vi "MTS_Main.vi"() -> ()   [LabVIEW 2010]
panel:
  out "Counts":u32[](array[numeric])
  in  "Autopoint-Auto Z":bool=TRUE
  in  "psf width [um]":dbl=0.7
  out "Last Image File No":i32
  out "NxtAutMesPoint":i32
  out "Auto Measure Points":i32
  out "Pattern":dbl[][](array[numeric])
  out "Active pt3":path
  in  "Axis":enum32{"x-y", "x-z", "y-z"}(ring)
  in  "Save Files":bool=TRUE
  out "Intensity (a.u.)":dbl=1.0 format="%.02f"
  out "Detector2":bool
  out "Detector1":bool
  out "Excitation":bool
  in  "Measurement Time (ms)":i32=60000 min=10
  in  "Open MSW":bool
  in  "New MSW":bool
  out "Workspace":path
  in  "WS File Tree":string(tree)
  out "Stop Measurement":bool
  in  "Learning loop":bool=TRUE
  in  "ShowTab":T1(tab)=enum."TCSPC Histogram"
  out "Video":u8[][](graph)
  in  "Find Mols":bool
  out "Image":i32[][](graph)
  in  "Save Color Image":bool
  out "Auto Meas Progress":i32(slide) caption="Point 1 / 1" scale=0.0..1.0
  out "AM image":T2(plugin-control)
  in  "Auto Meas":bool
  in  "Auto Measurement Time (ms)":i32=10000 caption="Measurement Time (ms)" min=10
  out "Histogram":i32[][](graph)
  out "Trace":i32[][](graph)
  out "FiFo Overrun":bool
  in  "SCANNER EMERGENCY":bool
  out "Measure. time [s]":i32
  in  "Scanner Divider":i32=2 min=1 max=10
  out "y":dbl format="%.1f nm"
  out "x":dbl format="%.1f nm"
  in  "x-Pixel":u16=100
  in  "y-Pixel":u16=100
  in  "Picture size":dbl=50.0 min=0.1 max=200.0 format="%1.1f um"
  in  "Picture size 2":dbl=50.0 min=0.1 max=200.0 format="%1.1f um"
  in  "Z-Position":dbl=50.0 caption="Z" min=0.0 max=200.0 format="%1.3f um"
  in  "Y-Position":dbl=50.0 caption="Y" min=0.0 max=200.0 format="%1.3f um"
  in  "X-Position":dbl=50.0 caption="X" min=0.0 max=200.0 format="%1.3f um"
  out "Do Measurement":T3(ring)
  in  "Point Measurement":bool
  in  "Aquire Image":bool
  in  "Settings":bool
  in  "PI E710 Port":u16(ring) items=["COM1", "COM2", "COM3", "COM4", "COM5", "COM6", "COM7", "COM8", "COM9"]
  in  "Move Stage":bool
  out "MeasRunig":bool
  in  "Stop Program":bool
  out "Global Stop":bool
  # "Workspace"
  # "Shutter:"
  # "Image Scan Settings"
  # "Point Measurement Settings"
  # "upper left corner/ Point Position"
  # "Auto Measurement Settings"
  # "Pixelsize"
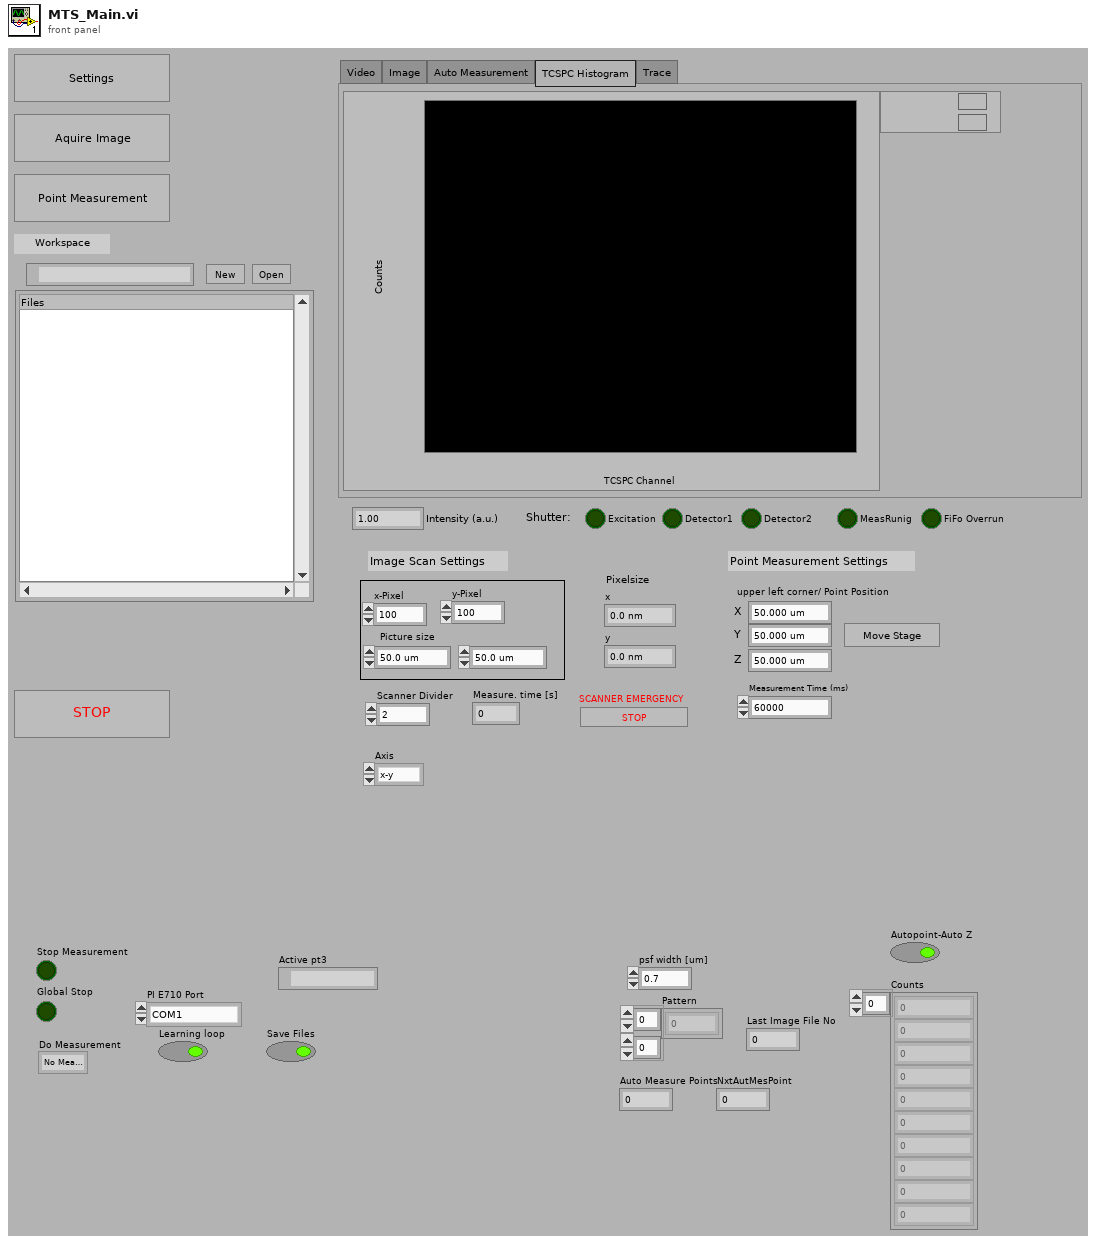
[diagram p1: front panel]
types:
  T1 = enum32{"Video", "Image", "Auto Measurement", "TCSPC Histogram", "Trace"}
  T2 = typedef "IMAQ Image.ctl" = refnum<image>
  T3 = enum16{"No Measurement", "Aquire Image", "Point Measurement", "Multi Measurement", "Save Color Image", "Find Single Mol.", "Auto Measurement Control", "Auto Point"}
  T4 = enum16{"CAN_Baud_1M", "CAN_BAUD_500K", "CAN_BAUD_250K", "CAN_BAUD_125K", "CAN_BAUD_100K", "CAN_BAUD_50K", "CAN_BAUD_20K", "CAN_BAUD_10K", "CAN_BAUD_5K", "User"}
  T5 = enum16{"No Measurement", "Aquire Image", "Point Measurement", "Multi Measurement"}
  T6 = typedef "Image Type" = u32
  T7 = cluster{"Height":u32, "Width":u32, "Pixel Depth":u32}
  T8 = cluster{"Dev":i32, "SerNo":string, "HW_Model":string, "HW_Version":string}[]
  T9 = enum32{"Video", "Image", "TCSPC Histogram", "Trace"}
  T10 = cluster{"ID":u32, "MSG type":enum8{"STD, NO RTR", "STD,RTR", "XTD, NO RTR", "XTD, RTR"}, "LEN":u8, "DATA":u8[]}
  T11 = enum16{"No Measurement", "Aquire Image", "Point Measurement", "Multi Measurement", "Save Color Image"}
  T12 = enum16{"No Measurement", "Aquire Image", "Point Measurement", "Multi Measurement", "Save Color Image", "Find Single Mol."}
  T13 = enum16{"Get (Default)", "Set Workspace", "Append File", "Change Comment"}
  T14 = enum16{"unknown", "pt3 File", "png Image", "bmp Image"}
  T15 = cluster{"File No":i32, "File Path":path, "Parent File":i32, "File Type":enum16{"unknown", "pt3 File", "png Image", "bmp Image"}, "Measurement Type":enum16{"not a pt3 File", "Image File", "Point Measurement", "Auto Point"}, "Upper Left":cluster{"x-Position":dbl, "y-Position":dbl, "z-Position":dbl}, "Pixels":i32[], "Picture Size":dbl[], "Scan Axis":enum32{"x-y", "x-z", "y-z"}}[]
  T16 = typedef "LVPoint32TypeDef.ctl" = cluster{"Horizontal":i32, "Vertical":i32}
  T17 = cluster{"Shift":bool, "Ctrl":bool, "Alt":bool, "Cmd":bool, "Opt":bool}
  T18 = cluster{"File No":i32, "File Path":path, "Parent File":i32, "File Type":enum16{"unknown", "pt3 File", "png Image", "bmp Image"}, "Measurement Type":enum16{"not a pt3 File", "Image File", "Point Measurement", "Auto Point"}, "Upper Left":cluster{"x-Position":dbl, "y-Position":dbl, "z-Position":dbl}, "Pixels":i32[], "Picture Size":dbl[], "Scan Axis":enum32{"x-y", "x-z", "y-z"}}
  T19 = enum16{"not a pt3 File", "Image File", "Point Measurement", "Auto Point"}
  T20 = cluster{"x-Position":dbl, "y-Position":dbl, "z-Position":dbl}
  T21 = cluster{"ID":u32, "MSG type":enum8{"STD, NO RTR", "STD,RTR", "XTD, NO RTR", "XTD, RTR"}, "LEN":u8, "Data":u8[]}
  T22 = cluster{"X-Position":dbl, "Y-Position":dbl, "Z-Position":dbl}
  T23 = cluster{"Dimensions":i32, "Time Per Pixel [ms]":dbl, "Acceleration":i32, "Pattern":i32, "X0":sgl, "Y0":sgl, "PixX":i32, "PixY":i32, "PixResol":sgl, "TStartTo":sgl, "TStoptTo":sgl, "TStartFro":sgl, "TStopFro":sgl}
  T24 = cluster{"Picture Size":dbl[], "Pixels":i32[], "Upper Left":cluster{"x-Position":dbl, "y-Position":dbl, "z-Position":dbl}}
  T25 = cluster{"Dev":i32, "SerNo":string, "HW_Model":string, "HW_Version":string}
  T26 = cluster{"Comment":string, "RangeNo":i32, "Offset":i32, "AcquisitionTime (ms)":i32, "HardwareSerial":i32, "SyncDivider":i32, "Resolution (ns)":sgl, "CFD Settings":cluster{"Ch0 Level":i32, "Ch0 ZeroX":i32, "Ch1 Level":i32, "Ch1 ZeroX":i32}, "InpRate0":i32, "InpRate1":i32}
  T27 = cluster{"Ident":string, "Format Version":string, "Creator Name":string, "Creator Version":string, "File Time":string, "Comment":string, "RangeNo":i32, "Offset":i32, "AcquisitionTime (ms)":i32, "HardwareSerial":i32, "SyncDivider":i32, "Resolution (ns)":sgl, "CFD Settings":cluster{"Ch0 Level":i32, "Ch0 ZeroX":i32, "Ch1 Level":i32, "Ch1 ZeroX":i32}, "InpRate0":i32, "InpRate1":i32}
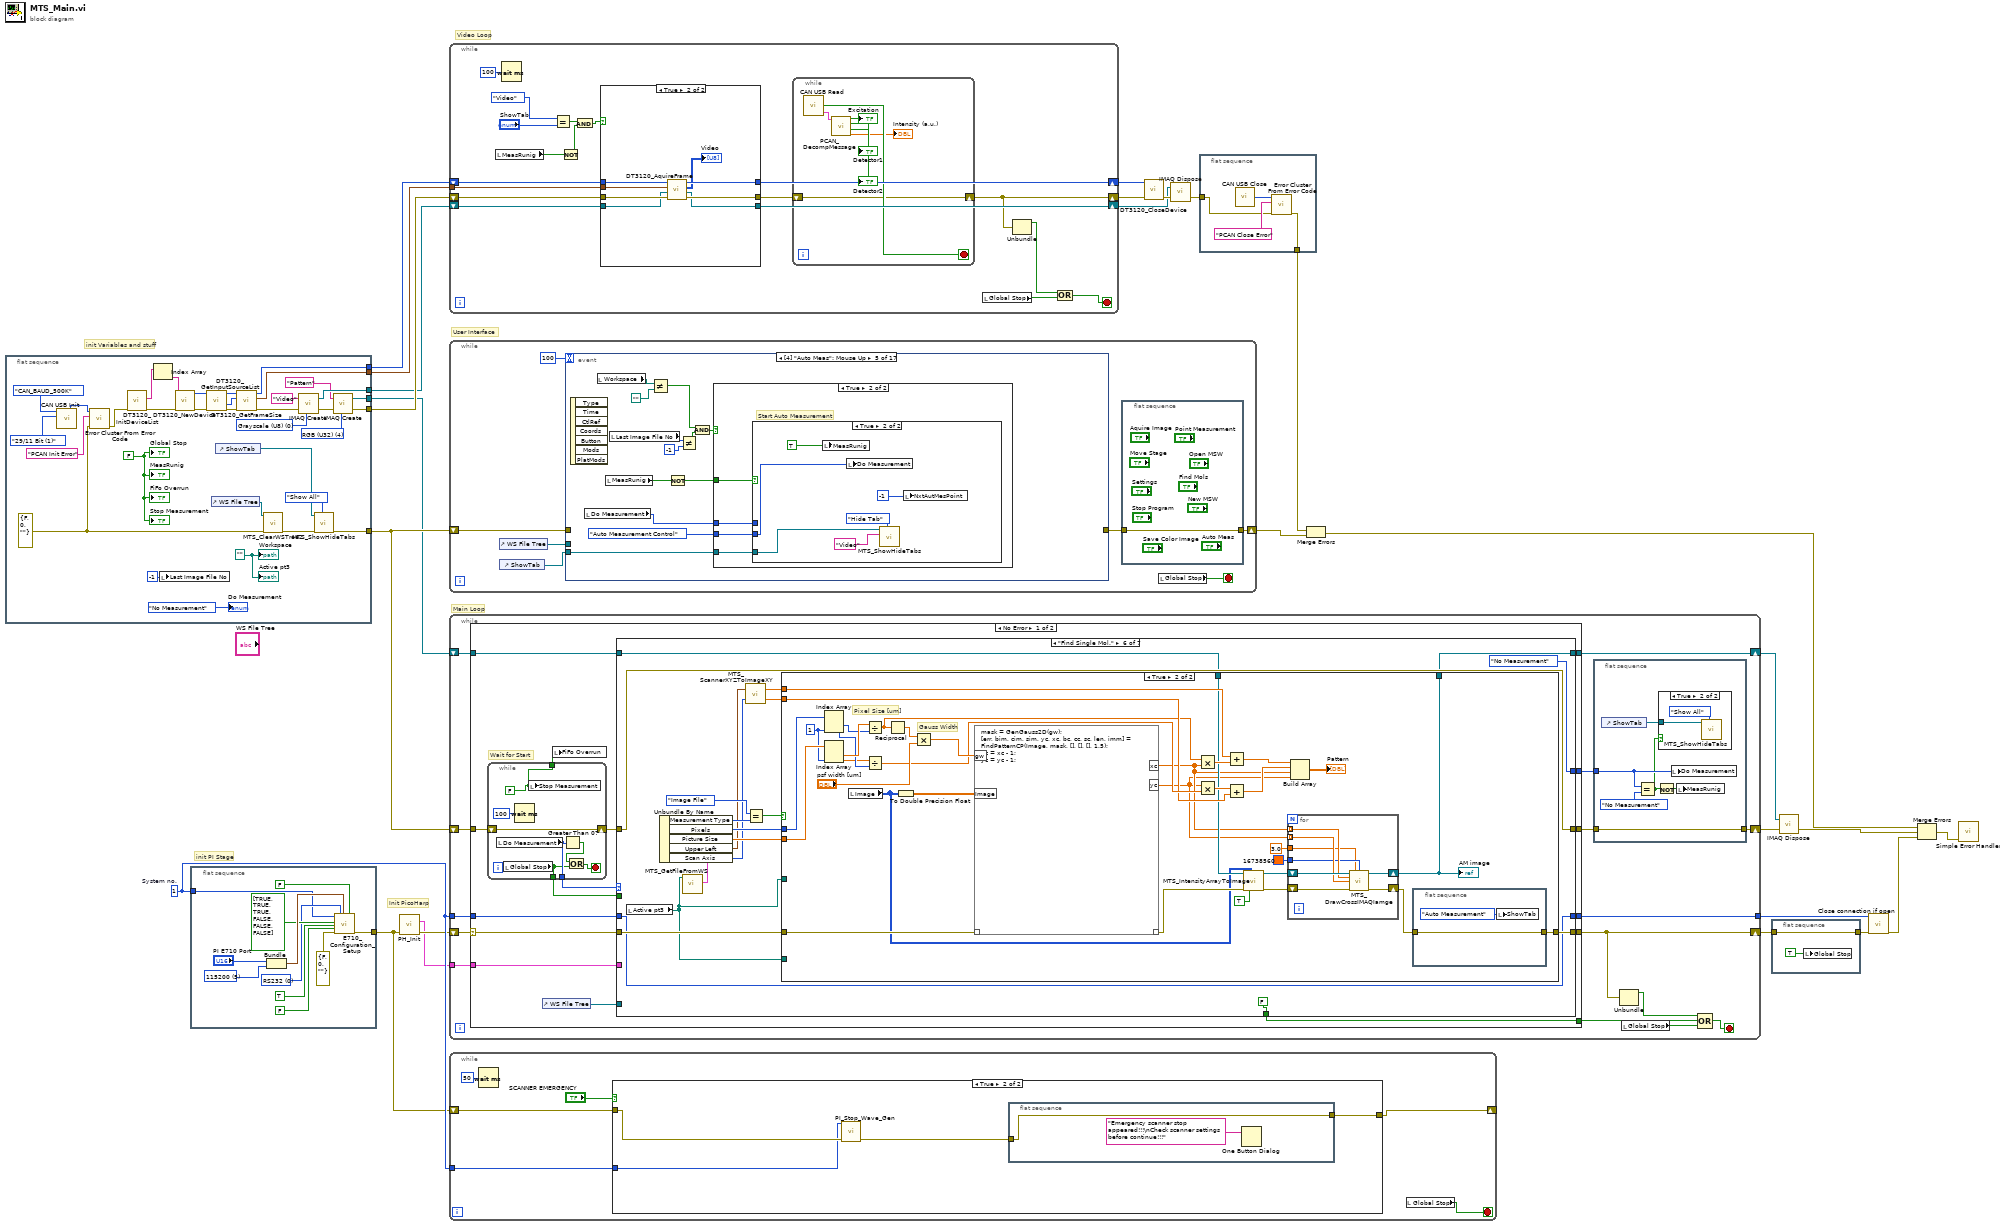
[diagram p0: block diagram]
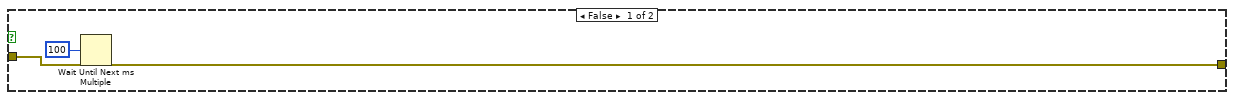
[diagram p3: hidden frame]
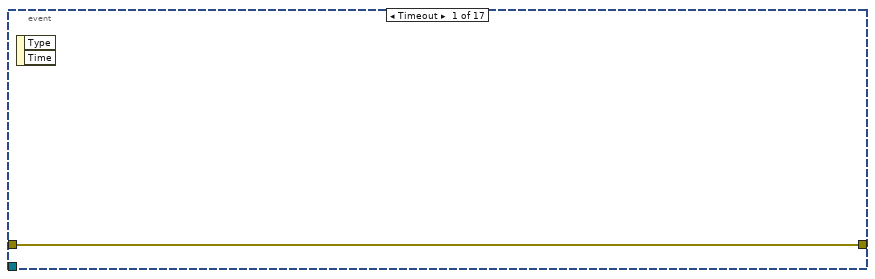
[diagram p4: hidden frame]
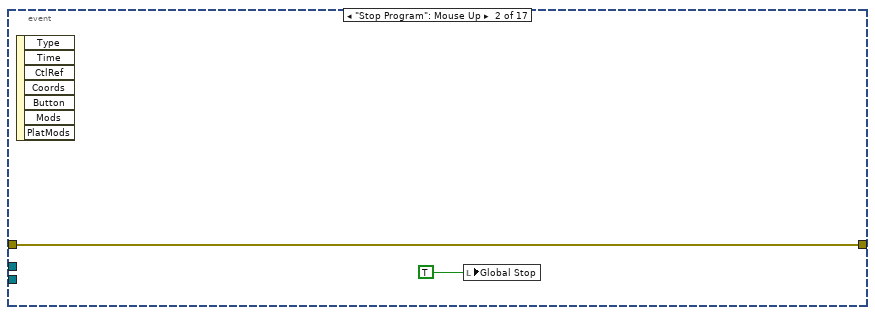
[diagram p5: hidden frame]
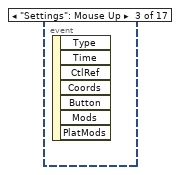
[diagram p6: hidden frame]
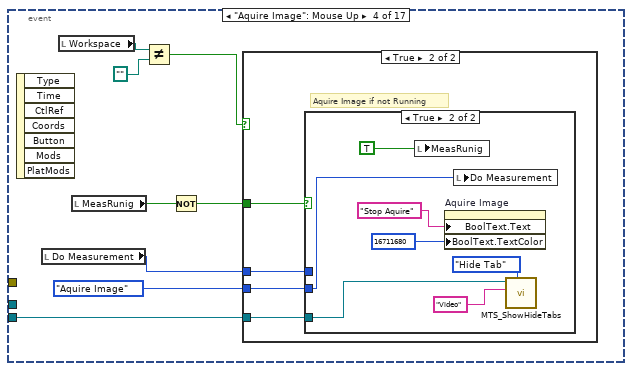
[diagram p7: hidden frame]
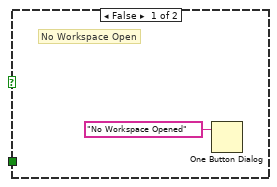
[diagram p8: hidden frame]
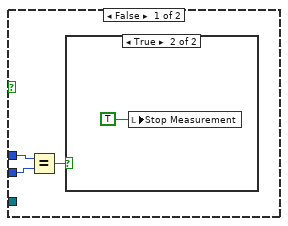
[diagram p9: hidden frame]
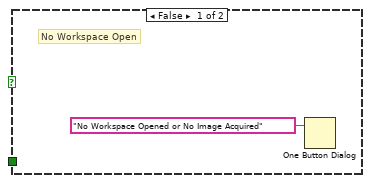
[diagram p11: hidden frame]
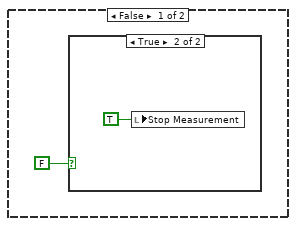
[diagram p12: hidden frame]
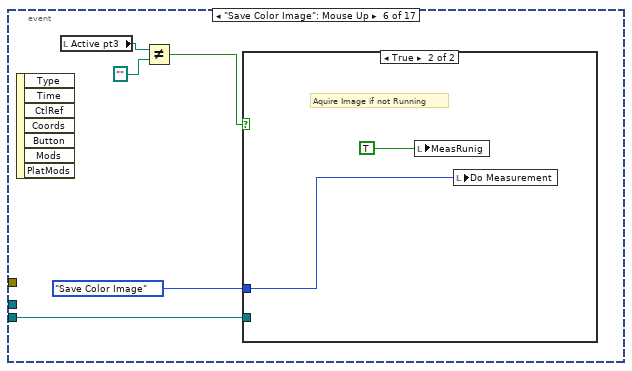
[diagram p14: hidden frame]
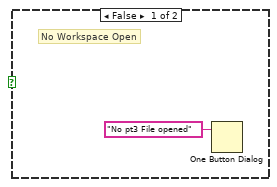
[diagram p15: hidden frame]
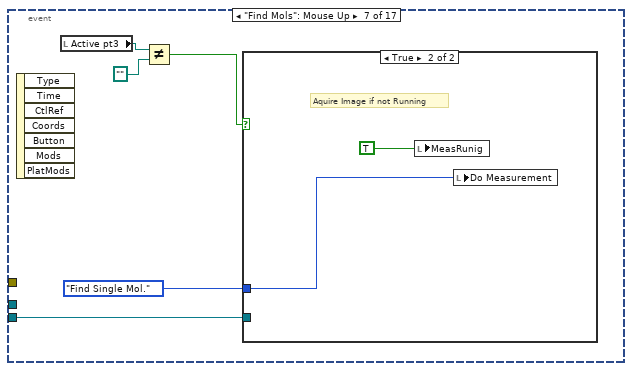
[diagram p16: hidden frame]
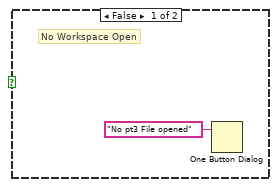
[diagram p17: hidden frame]
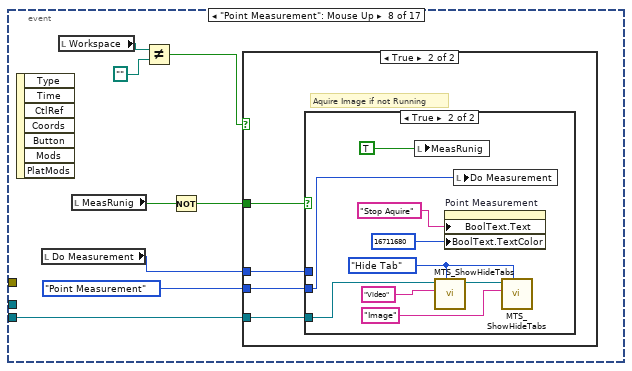
[diagram p18: hidden frame]
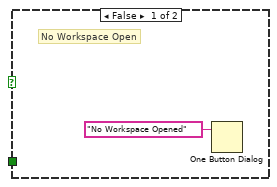
[diagram p19: hidden frame]
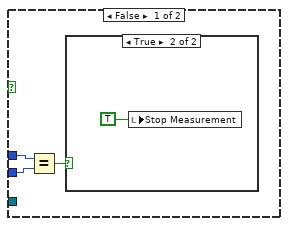
[diagram p20: hidden frame]
diagram:
  w22 = 1  # System no.
  # "Video Loop"
  # "Init PicoHarp"
  # "init Variables and stuff"
  # "User Interface"
  # "init PI Stage"
  # "Main Loop"
  n1 = flat-sequence {
    tunnel: [w43] -> w23
    tunnel: [w32] -> w16
    tunnel: [w50] -> w14
    tunnel: [w47] -> w10
    tunnel: [w31] -> w9
    tunnel: [w28] -> w1
    frame #0 {
      w29 = T6 4 items=["Grayscale (U8)", "Grayscale (I16)", "Grayscale (SGL)", "Complex (CSG)", "RGB (U32)", "HSL (U32)", "RGB (U64)", "Grayscale (U16)"] ("Image Type")
      w48 = T6 0 items=["Grayscale (U8)", "Grayscale (I16)", "Grayscale (SGL)", "Complex (CSG)", "RGB (U32)", "HSL (U32)", "RGB (U64)", "Grayscale (U16)"] ("Image Type")
      w34 = path ""
      w37 = errorcluster {"status"=FALSE, "code"=0, "source"=""} ("error in")
      w59 = FALSE ("Global Stop")
      n2 = call "CAN USB Init.vi"("CAN Msg Type"=enum16{"11 Bit (0)", "29/11 Bit (1)"}."29/11 Bit (1)", "BTR0BTR1"=T4."CAN_BAUD_500K") -> ("Error Number"=w38:u32)  [unwired: 7 in, 2 out]
      n3 = call <vilib>:"Error Cluster From Error Code.vi"("error in (no error)"=w37, "error message (\"\")"="PCAN Init Error" ("error message (\"\")"), "error code (0)"=w38) -> ("error out"=w36:errorcluster)  [unwired: 6 in]
      n4 = call "DT3120_InitDeviceList.vi"("error in (no error)"=w36) -> ("error out"=w57:errorcluster, "Alias List"=w58:string[])  [unwired: 9 out]
      n5 = Index Array(array=w58) -> (element=w56:string)  [unwired: 1 in]
      n6 = local write "Last Image File No"(-1 ("Last Image File No")) -> ()
      n7 = call "DT3120_NewDevice.vi"("error in (no error)"=w57, "Alias"=w56) -> ("error out"=w52:errorcluster, "DevId"=w51:i32)  [unwired: 8 out]
      n8 = call "DT3120_GetInputSourceList.vi"("error in (no error)"=w52, "DevId"=w51) -> ("error out"=w55:errorcluster, "Active Source"=w54:u16, "DevId (dup)"=w53:i32)  [unwired: 7 out]
      n9 = control-ref of="WS File Tree"() -> (w45:refnum<vi>)
      n10 = control-ref of="ShowTab"() -> (w42:refnum<vi>)
      n11 = call "DT3120_GetFrameSize.vi"("error in (no error)"=w55, "Source"=w54, "DevId"=w53) -> ("error out"=w49:errorcluster, "Frame Size"=w47:T7, "DevId (dup)"=w50:i32)  [unwired: 6 in]
      n12 = call "MTS_ClearWSTree2.vi"("error in"=w37, "Tree Refnum"=w45) -> ("error out"=w44:errorcluster)  [unwired: 8 in, 1 out]
      n13 = call "IMAQ Create"("Image Name"="Video", "Image Type"=w48, "error in (no error)"=w49) -> ("New Image"=w31:T2, "error out"=w33:errorcluster)  [unwired: 2 in]
      n14 = call "MTS_ShowHideTabs.vi"("Action"=enum16{"Show All", "Hide Tab", "Show Tab"}."Show All", "error in (no error)"=w44, "ShowTab"=w42) -> ("error out"=w43:errorcluster)  [unwired: 7 in, 1 out]
      n15 = call "IMAQ Create"("Image Name"="Pattern", "Image Type"=w29, "error in (no error)"=w33) -> ("New Image"=w28:T2, "error out"=w32:errorcluster)  [unwired: 2 in]
      "Global Stop" <- w59
      "MeasRunig" <- w59
      "Do Measurement" <- T5."No Measurement" ("Do Measurement")
      "FiFo Overrun" <- w59
      "Stop Measurement" <- w59
      "Workspace" <- w34
      "Active pt3" <- w34
    }
  }
  n16 = flat-sequence {
    tunnel: [w63] -> w21
    tunnel: w22 -> [w62]
    frame #0 {
      w70 = u16 5 items=["9600", "14400", "19200", "38400", "57600", "115200"] ("Baudrate")
      w65 = u16 0 items=["RS232", "GPIB"] ("Interface")
      n17 = Bundle("PI E710 Port"="PI E710 Port", "Baudrate"=w70) -> (w71:cluster{"PI E710 Port":u16, "Baudrate":u16})  [unwired: 1 out]
      n18 = call <userlib>:"E710_Configuration_Setup.vi"("System no."=w62, "Are stages connected?"=bool[] [TRUE, TRUE, TRUE, FALSE, FALSE, FALSE], "Change servo \nstatus to ON?"=TRUE ("Change servo \nstatus to ON?"), "Perform autozero?"=FALSE ("All axes?"), "error in"=errorcluster {"status"=FALSE, "code"=0, "source"=""}, "Interface"=w65, "RS232 settings"=w71, "Move to middle?"=FALSE) -> ("error out"=w63:errorcluster)  [unwired: 4 in, 7 out]
    }
  }
  n19 = call "PH_Init.vi"("error in (no error)"=w21) -> ("Device List"=w19:T8, "error out"=w20:errorcluster)  [unwired: 12 in, 1 out]
  n20 = while {
    shift-right: [w72] -> w15
    shift-left: w16 -> [w86]
    shift-right: [w79] -> w13
    shift-left: w14 -> [w80]
    tunnel: w10 -> [w81]
    shift-right: [w78] -> w7
    shift-left: w9 -> [w82]
    stop <- w85 stop-if-true
    n21 = local read "MeasRunig"() -> (w77:bool)
    n22 = Wait (ms)(milliseconds to wait=u32 100) -> ()  [unwired: 1 out]
    n23 = Equal?(x=T9."Video" ("ShowTab"), y="ShowTab") -> (x = y?=w76:bool)
    n24 = Not(x=w77) -> (.not. x?=w74:bool)
    n25 = And(x=w76, y=w74) -> (x .and. y?=w75:bool)
    n26 = case shown="True" w75 {
      tunnel: w86 -> [w99 w107]
      tunnel: [w99 w106] -> w73
      tunnel: w82 -> [w97 w105]
      tunnel: w81 -> [_ w104]
      tunnel: w80 -> [w98 w103]
      tunnel: [w98 w102] -> w79
      tunnel: [w97 w101] -> w78
      frame False {
      }
      frame True {
        n27 = call "DT3120_AquireFrame.vi"("error in (no error)"=w107, "Image"=w105, "Frame Size"=w104, "DevId"=w103) -> ("error out"=w106:errorcluster, "Image Out"=w101:T2, "Frame"=→"Video":u8[][], "DevId (dup)"=w102:i32)  [unwired: 4 in]
      }
    }
    n28 = while {
      shift-right: [w91] -> w72
      shift-left: w73 -> [w91]
      stop <- w96 stop-if-true
      n29 = call "CAN USB Read.vi"() -> ("RcvQueueEmpty"=w96:bool, "CAN_Message out"=w95:T10)  [unwired: 1 in, 1 out]
      n30 = call "PCAN_DecompMessage.vi"("CAN_Message out"=w95) -> ("Intensity (a.u.)"=→"Intensity (a.u.)":dbl, "Detector2 Shutter Open?"=→"Detector2":bool, "Detector1 Shutter Open?"=→"Detector1":bool, "Excitation Shutter Open?"=→"Excitation":bool)  [unwired: 7 in]
    }
    n31 = local read "Global Stop"() -> (w84:bool)
    n32 = Unbundle(w72) -> ("status"=w83:bool)  [unwired: 2 out]
    n33 = Compound Arithmetic op=OR(w83, w84) -> (w85:bool)
  }
  n34 = while {
    shift-right: [w112] -> w12
    shift-left: w23 -> [w113]
    stop <- w110 stop-if-true
    n35 = control-ref of="WS File Tree"() -> (w109:refnum<vi>)
    n36 = control-ref of="ShowTab"() -> (w108:refnum<vi>)
    n37 = event shown="[4] \"Auto Meas\": Mouse Up" {
      selector: _ -> [_ _ _ _ _ _ _ _ _ _ _ _ _ _ _ _ _]
      dyn-events: _ -> [_ _ _ _ _ _ _ _ _ _ _ _ _ _ _ _ _]
      timeout: 100 -> [_ _ _ _ _ _ _ _ _ _ _ _ _ _ _ _ _]
      tunnel: w113 -> [w116 w118 _ _ _ _ _ _ _ w227 w263 _ w315 _ _ _ _]
      tunnel: [w116 w118 _ _ _ _ _ _ _ w225 w260 _ w314 _ _ _ _] -> w111
      tunnel: w109 -> [_ _ _ _ _ _ _ _ _ w229 w264 _ _ _ _ _ _]
      tunnel: w108 -> [_ _ _ w119 w149 w168 w176 w184 w210 _ _ _ _ _ _ _ _]
      event Timeout {
        n38 = event-data() -> ()  [unwired: 1 in, 2 out]
      }
      event "Stop Program": Mouse Up {
        n39 = event-data() -> ()  [unwired: 1 in, 7 out]
        n40 = local write "Global Stop"(TRUE ("Global Stop")) -> ()
      }
      event "Settings": Mouse Up {
        n41 = event-data() -> ()  [unwired: 1 in, 7 out]
      }
      event "Aquire Image": Mouse Up {
        n42 = event-data() -> ()  [unwired: 1 in, 7 out]
        n43 = local read "Do Measurement"() -> (w123:T3)
        n44 = local read "Workspace"() -> (w122:path)
        n45 = local read "MeasRunig"() -> (w126:bool)
        n46 = Not Equal?(x=w122, y=path "") -> (x != y?=w120:bool)
        n47 = Not(x=w126) -> (.not. x?=w125:bool)
        n48 = case shown="True" w120 {
          tunnel: w125 -> [_ w131]
          tunnel: T11."Aquire Image" ("Do Measurement") -> [_ w130]
          tunnel: w123 -> [_ w129]
          tunnel: w119 -> [_ w128]
          frame False {
            # "No Workspace Open"
            n49 = One Button Dialog(message="No Workspace Opened") -> ()  [unwired: 1 in, 1 out]
          }
          frame True {
            # "Aquire Image if not Running"
            n50 = case shown="True" w131 {
              tunnel: w130 -> [w133 w140]
              tunnel: w129 -> [w134 _]
              tunnel: w128 -> [_ w136]
              frame False {
                n51 = Equal?(x=w134, y=w133) -> (x = y?=w132:bool)
                n52 = case shown="True" w132 {
                  frame False {
                  }
                  frame True {
                    n53 = local write "Stop Measurement"(TRUE ("Stop Measurement")) -> ()
                  }
                }
              }
              frame True {
                n54 = local write "MeasRunig"(TRUE ("Measurement Running")) -> ()
                n55 = property on="Aquire Image" class="Bool"("BoolText.Text"="Stop Aquire" ("Caption.Text"), "BoolText.TextColor"=u32 16711680 ("Boolean Text.Colors:FG Color")) -> ()  [unwired: 2 in, 2 out]
                n56 = local write "Do Measurement"(w140) -> ()
                n57 = call "MTS_ShowHideTabs.vi"("Action"=enum16{"Show All", "Hide Tab", "Show Tab"}."Hide Tab", "Tab Caption"="Video", "ShowTab"=w136) -> ()  [unwired: 7 in, 2 out]
              }
            }
          }
        }
      }
      event "Auto Meas": Mouse Up {
        n58 = event-data() -> ()  [unwired: 1 in, 7 out]
        n59 = local read "Do Measurement"() -> (w152:T3)
        n60 = local read "Workspace"() -> (w151:path)
        n61 = local read "MeasRunig"() -> (w154:bool)
        n62 = local read "Last Image File No"() -> (w147:i32)
        n63 = Not Equal?(x=w151, y=path "") -> (x != y?=w145:bool)
        n64 = Not(x=w154) -> (.not. x?=w153:bool)
        n65 = Not Equal?(x=w147, y=-1) -> (x != y?=w144:bool)
        n66 = And(x=w145, y=w144) -> (x .and. y?=w143:bool)
        n67 = case shown="True" w143 {
          tunnel: w153 -> [_ w159]
          tunnel: T3."Auto Measurement Control" ("Do Measurement") -> [_ w158]
          tunnel: w152 -> [_ w157]
          tunnel: w149 -> [_ w156]
          frame False {
            # "No Workspace Open"
            n68 = One Button Dialog(message="No Workspace Opened or No Image Acquired") -> ()  [unwired: 1 in, 1 out]
          }
          frame True {
            # "Start Auto Measurement"
            n69 = case shown="True" w159 {
              tunnel: w158 -> [_ w166]
              tunnel: w157 -> [_ _]
              tunnel: w156 -> [_ w163]
              frame False {
                n70 = case shown="True" FALSE {
                  frame False {
                  }
                  frame True {
                    n71 = local write "Stop Measurement"(TRUE ("Stop Measurement")) -> ()
                  }
                }
              }
              frame True {
                n72 = local write "MeasRunig"(TRUE ("Measurement Running")) -> ()
                n73 = local write "Do Measurement"(w166) -> ()
                n74 = call "MTS_ShowHideTabs.vi"("Action"=enum16{"Show All", "Hide Tab", "Show Tab"}."Hide Tab", "Tab Caption"="Video", "ShowTab"=w163) -> ()  [unwired: 7 in, 2 out]
                n75 = local write "NxtAutMesPoint"(-1 ("Next Auto Measure Point")) -> ()
              }
            }
          }
        }
      }
      event "Save Color Image": Mouse Up {
        n76 = event-data() -> ()  [unwired: 1 in, 7 out]
        n77 = local read "Active pt3"() -> (w171:path)
        n78 = Not Equal?(x=w171, y=path "") -> (x != y?=w169:bool)
        n79 = case shown="True" w169 {
          tunnel: T12."Save Color Image" ("Do Measurement") -> [_ w175]
          tunnel: w168 -> [_ _]
          frame False {
            # "No Workspace Open"
            n80 = One Button Dialog(message="No pt3 File opened") -> ()  [unwired: 1 in, 1 out]
          }
          frame True {
            # "Aquire Image if not Running"
            n81 = local write "MeasRunig"(TRUE ("Measurement Running")) -> ()
            n82 = local write "Do Measurement"(w175) -> ()
          }
        }
      }
      event "Find Mols": Mouse Up {
        n83 = event-data() -> ()  [unwired: 1 in, 7 out]
        n84 = local read "Active pt3"() -> (w179:path)
        n85 = Not Equal?(x=w179, y=path "") -> (x != y?=w177:bool)
        n86 = case shown="True" w177 {
          tunnel: T12."Find Single Mol." ("Do Measurement") -> [_ w183]
          tunnel: w176 -> [_ _]
          frame False {
            # "No Workspace Open"
            n87 = One Button Dialog(message="No pt3 File opened") -> ()  [unwired: 1 in, 1 out]
          }
          frame True {
            # "Aquire Image if not Running"
            n88 = local write "MeasRunig"(TRUE ("Measurement Running")) -> ()
            n89 = local write "Do Measurement"(w183) -> ()
          }
        }
      }
      event "Point Measurement": Mouse Up {
        n90 = event-data() -> ()  [unwired: 1 in, 7 out]
        n91 = local read "Do Measurement"() -> (w188:T3)
        n92 = local read "Workspace"() -> (w187:path)
        n93 = local read "MeasRunig"() -> (w191:bool)
        n94 = Not Equal?(x=w187, y=path "") -> (x != y?=w185:bool)
        n95 = Not(x=w191) -> (.not. x?=w190:bool)
        n96 = case shown="True" w185 {
          tunnel: w190 -> [_ w196]
          tunnel: T11."Point Measurement" ("Do Measurement") -> [_ w195]
          tunnel: w188 -> [_ w194]
          tunnel: w184 -> [_ w193]
          frame False {
            # "No Workspace Open"
            n97 = One Button Dialog(message="No Workspace Opened") -> ()  [unwired: 1 in, 1 out]
          }
          frame True {
            # "Aquire Image if not Running"
            n98 = case shown="True" w196 {
              tunnel: w195 -> [w198 w207]
              tunnel: w194 -> [w199 _]
              tunnel: w193 -> [_ w204]
              frame False {
                n99 = Equal?(x=w199, y=w198) -> (x = y?=w197:bool)
                n100 = case shown="True" w197 {
                  frame False {
                  }
                  frame True {
                    n101 = local write "Stop Measurement"(TRUE ("Stop Measurement")) -> ()
                  }
                }
              }
              frame True {
                w201 = enum16{"Show All", "Hide Tab", "Show Tab"}."Hide Tab" ("Action")
                n102 = local write "MeasRunig"(TRUE ("Measurement Running")) -> ()
                n103 = call "MTS_ShowHideTabs.vi"("Action"=w201, "Tab Caption"="Video", "ShowTab"=w204) -> ("ShowTab (dup)"=w203:refnum<vi>)  [unwired: 7 in, 1 out]
                n104 = property on="Point Measurement" class="Bool"("BoolText.Text"="Stop Aquire" ("Caption.Text"), "BoolText.TextColor"=u32 16711680 ("Boolean Text.Colors:FG Color")) -> ()  [unwired: 2 in, 2 out]
                n105 = local write "Do Measurement"(w207) -> ()
                n106 = call "MTS_ShowHideTabs.vi"("Action"=w201, "Tab Caption"="Image", "ShowTab"=w203) -> ()  [unwired: 7 in, 2 out]
              }
            }
          }
        }
      }
      event "Move Stage": Mouse Up {
        n107 = event-data() -> ()  [unwired: 1 in, 7 out]
        n108 = local read "Do Measurement"() -> (w214:T3)
        n109 = local read "Workspace"() -> (w213:path)
        n110 = local read "MeasRunig"() -> (w217:bool)
        n111 = Not Equal?(x=w213, y=path "") -> (x != y?=w211:bool)
        n112 = Not(x=w217) -> (.not. x?=w216:bool)
        n113 = case shown="True" w211 {
          tunnel: w216 -> [_ w222]
          tunnel: T11."Multi Measurement" ("Do Measurement") -> [_ w221]
          tunnel: w214 -> [_ w220]
          tunnel: w210 -> [_ w219]
          frame False {
            # "No Workspace Open"
            n114 = One Button Dialog(message="No Workspace Opened") -> ()  [unwired: 1 in, 1 out]
          }
          frame True {
            # "Aquire Image if not Running"
            n115 = case shown="True" w222 {
              tunnel: w221 -> [_ w223]
              tunnel: w220 -> [_ _]
              tunnel: w219 -> [_ _]
              frame False {
              }
              frame True {
                n116 = local write "MeasRunig"(TRUE ("Measurement Running")) -> ()
                n117 = local write "Do Measurement"(w223) -> ()
              }
            }
          }
        }
      }
      event "New MSW": Mouse Up {
        # "Default Name"
        n118 = event-data() -> ()  [unwired: 1 in, 7 out]
        n119 = flat-sequence {
          tunnel: [w245] -> w228
          tunnel: w227 -> [w245]
          frame #0 {
            n120 = local write "MeasRunig"(TRUE ("MeasRunig")) -> ()
          }
        }
        n121 = Get Date/Time In Seconds() -> (seconds since 1Jan1904=w242:timestamp)
        n122 = Format Date/Time String(time format string (%c)="%Y-%m-%d", seconds (now)=w242) -> (date/time string=w240:string)  [unwired: 1 out]
        n123 = Concatenate Strings(w240, ".msw" ("string")) -> (w238:string)
        n124 = call "File Dialog"("start path"=path "E:/", "prompt"="Create New Workspace", "button label"="Create", "default name"=w238, "error in"=w228, "pattern (all files)"="*.msw", "pattern label"="MT Scan Workspace") -> ("selected path"=w232:path, "cancelled"=w233:bool, "error out"=w231:errorcluster)  [unwired: 5 in, 1 out]
        n125 = case shown="False" w233 {
          tunnel: w232 -> [w251 _]
          tunnel: w231 -> [w257 w259]
          tunnel: [w249 w258] -> w226
          tunnel: w229 -> [w247 _]
          frame False {
            # "Create Empty Workspace"
            n126 = local write "Workspace"(w251) -> ()
            n127 = call "MTS_CreateWriteMSW.vi"("Rewrite"=TRUE, "error in (no error)"=w257, "Workspace Path"=w251) -> ("error out"=w250:errorcluster, "Created"=w254:string, "Comment (dup)"=w253:string, "Files in Workspace (dup)"=w252:T15)  [unwired: 5 in]
            n128 = call "MTS_Workspace.vi"("Workspace"=w251, "Operation"=T13."Set Workspace", "Created in"=w254, "New Comment"=w253, "Files in Workspace in"=w252) -> ("Files in Workspace"=w248:T15)  [unwired: 3 in, 3 out]
            n129 = call "MTS_BuildWSTree.vi"("error in"=w250, "Files in Workspace"=w248, "Tree Refnum"=w247) -> ("error out"=w249:errorcluster)  [unwired: 7 in, 1 out]
          }
          frame True {
            n130 = call <vilib>:"Clear Errors.vi"("error in (no error)"=w259) -> ("error out"=w258:errorcluster)  [unwired: 6 in]
          }
        }
        n131 = flat-sequence {
          tunnel: w226 -> [w243]
          tunnel: [w243] -> w225
          frame #0 {
            n132 = local write "MeasRunig"(FALSE ("MeasRunig")) -> ()
          }
        }
      }
      event "Open MSW": Mouse Up {
        n133 = event-data() -> ()  [unwired: 1 in, 7 out]
        n134 = flat-sequence {
          tunnel: w263 -> [w275]
          tunnel: [w275] -> w262
          frame #0 {
            n135 = local write "MeasRunig"(TRUE ("MeasRunig")) -> ()
          }
        }
        n136 = call "File Dialog2"("start path"=path "E:/", "prompt"="Create New Workspace", "button label"="Open", "error in"=w262, "pattern (all files)"="*.msw", "pattern label"="MT Scan Workspace") -> ("selected path"=w267:path, "cancelled"=w268:bool, "error out"=w266:errorcluster)  [unwired: 6 in, 1 out]
        n137 = case shown="False" w268 {
          tunnel: w267 -> [w281 _]
          tunnel: w266 -> [w286 w288]
          tunnel: [w279 w287] -> w261
          tunnel: w264 -> [w277 _]
          frame False {
            # "Open Workspace"
            n138 = local write "Workspace"(w281) -> ()
            n139 = call "MTS_ReadMSW.vi"("error in (no error)"=w286, "Workspace Path"=w281) -> ("error out"=w280:errorcluster, "Created"=w284:string, "Comment"=w283:string, "Files in Workspace"=w282:T15)  [unwired: 6 in]
            n140 = call "MTS_Workspace.vi"("Workspace"=w281, "Operation"=T13."Set Workspace", "Created in"=w284, "New Comment"=w283, "Files in Workspace in"=w282) -> ("Files in Workspace"=w278:T15)  [unwired: 3 in, 3 out]
            n141 = call "MTS_BuildWSTree.vi"("error in"=w280, "Files in Workspace"=w278, "Tree Refnum"=w277) -> ("error out"=w279:errorcluster)  [unwired: 7 in, 1 out]
          }
          frame True {
            n142 = call <vilib>:"Clear Errors.vi"("error in (no error)"=w288) -> ("error out"=w287:errorcluster)  [unwired: 6 in]
          }
        }
        n143 = flat-sequence {
          tunnel: w261 -> [w273]
          tunnel: [w273] -> w260
          frame #0 {
            n144 = local write "MeasRunig"(FALSE ("MeasRunig")) -> ()
          }
        }
      }
      event "Image": Mouse Up {
        w291 = 100.0 ("y")
        n145 = event-data() -> ("Coords"=w303:T16, "PlatMods"=w304:T17)  [unwired: 1 in, 5 out]
        n146 = local read "Axis"() -> (w299:enum32{"x-y", "x-z", "y-z"})
        n147 = invoke on="Image" class="IntGraph (strict)" method="Map Coords To XY"("Coords"=w303) -> ("Map Coords To XY"=w300:bool, "XY"=w298:cluster{"X":dbl, "Y":dbl})  [unwired: 6 in, 5 out]
        n148 = Unbundle By Name(w304) -> ("Ctrl"=w301:bool)
        n149 = And(x=w300, y=w301) -> (x .and. y?=w302:bool)
        n150 = Unbundle(w298) -> ("X"=w297:dbl, "Y"=w294:dbl)
        n151 = Multiply(x=w297, y=w291) -> (x*y=w296:dbl)
        n152 = Multiply(x=w294, y=w291) -> (x*y=w293:dbl)
        n153 = Round To Nearest(number=w296) -> (nearest integer value=w295:dbl)
        n154 = Round To Nearest(number=w293) -> (nearest integer value=w292:dbl)
        n155 = Divide(x=w295, y=w291) -> (x/y=w290:dbl)
        n156 = Divide(x=w292, y=w291) -> (x/y=w289:dbl)
        n157 = case shown="True" w302 {
          tunnel: w299 -> [_ w307]
          tunnel: w290 -> [_ w306]
          tunnel: w289 -> [_ w305]
          frame False {
          }
          frame True {
            n158 = case shown="\"x-y\", Default" w307 {
              tunnel: w306 -> [w309 w311 w313]
              tunnel: w305 -> [w308 w310 w312]
              frame "x-y", Default {
                n159 = local write "X-Position"(w309) -> ()
                n160 = local write "Y-Position"(w308) -> ()
              }
              frame "x-z" {
                n161 = local write "X-Position"(w311) -> ()
                n162 = local write "Z-Position"(w310) -> ()
              }
              frame "y-z" {
                n163 = local write "Y-Position"(w313) -> ()
                n164 = local write "Z-Position"(w312) -> ()
              }
            }
          }
        }
      }
      event "WS File Tree": Value Change {
        n165 = event-data() -> ("NewVal"=w319:string)  [unwired: 1 in, 4 out]
        n166 = local read "Workspace"() -> (w316:path)
        n167 = Not Equal?(x=w316, y=path "") -> (x != y?=w317:bool)
        n168 = case shown="True" w317 {
          tunnel: w319 -> [_ w330]
          tunnel: w316 -> [_ w329]
          tunnel: w315 -> [w320 w328]
          tunnel: [w320 w327] -> w314
          frame False {
          }
          frame True {
            n169 = call "MTS_GetFileFromWS.vi"("Tree Label"=w330) -> ("File Header"=w326:T18, "File Found"=w325:bool)  [unwired: 9 in]
            n170 = Unbundle By Name(w326) -> ("File Type"=w324:T14)
            n171 = Equal?(x=w324, y=T14."pt3 File" ("File Type")) -> (x = y?=w322:bool)
            n172 = And(x=w325, y=w322) -> (x .and. y?=w321:bool)
            n173 = case shown="True" w321 {
              tunnel: w326 -> [_ w350]
              tunnel: w329 -> [_ w356]
              tunnel: w328 -> [w331 w351]
              tunnel: [w331 w338] -> w327
              frame False {
              }
              frame True {
                # "Image Intensity Array"
                n174 = Unbundle By Name(w350) -> ("Measurement Type"=w337:T19, "Pixels"=w335:i32[], "Picture Size"=w334:dbl[], "Upper Left"=w333:T20, "Scan Axis"=w332:enum32{"x-y", "x-z", "y-z"})
                n175 = Unbundle By Name(w350) -> ("File Path"=w355:path)
                n176 = Strip Path(path=w356) -> (stripped path=w354:path)  [unwired: 1 out]
                n177 = Strip Path(path=w355) -> (name=w353:string)  [unwired: 1 out]
                n178 = control-ref of="Image"() -> (w336:refnum<vi>)
                n179 = Build Path(base path=w354, name or relative path=w353) -> (appended path=w352:path)
                n180 = Index Array(array=w335, index #2=1 ("index")) -> (element #1=w347:i32, element #2=w346:i32)  [unwired: 1 in]
                n181 = local write "Active pt3"(w352) -> ()
                n182 = call "PT3_Open.vi"("error in"=w351, "File Path"=w352) -> ("error out"=w345:errorcluster, "refnum out"=w344:refnum<file>)  [unwired: 3 in, 5 out]
                n183 = Initialize Array(0 ("element"), w347, w346) -> (w343:i32[][])
                n184 = case shown="\"Image File\"" w337 {
                  tunnel: w345 -> [w363 w395]
                  tunnel: w344 -> [w370 w394]
                  tunnel: w343 -> [w369 w393]
                  tunnel: [w367 w392] -> w342
                  tunnel: [w366 w391] -> w341
                  tunnel: [w365 w390] -> w340
                  tunnel: [w364 w389] -> w339
                  tunnel: w336 -> [w361 _]
                  tunnel: w335 -> [w360 _]
                  tunnel: w334 -> [w359 _]
                  tunnel: w333 -> [w358 _]
                  tunnel: w332 -> [w357 _]
                  frame "Image File" {
                    n185 = call "MTS_SetGraphScales.vi"("Pixels"=w360, "Axis"=w357, "Picture Size"=w359, "error in (no error)"=w363, "Upper Left"=w358, "Image"=w361) -> ("error out"=w362:errorcluster)  [unwired: 5 in]
                    n186 = while {
                      tunnel: w370 -> [w385]
                      shift-right: [FALSE ("Start From Top")] -> _
                      shift-left: TRUE ("Start From Top") -> [w379]
                      shift-right: [w378] -> w364
                      shift-left: w362 -> [w374]
                      tunnel: [w377] -> w365
                      tunnel: [w376] -> w367
                      tunnel: [w375] -> w368
                      tunnel: w369 -> [w373]
                      tunnel: [w372] -> w366
                      stop <- w382 stop-if-true
                      n187 = call "PT3_Read.vi"("Start From Top"=w379, "error in"=w374, "Data count"=10000, "refnum in"=w385) -> ("error out"=w378:errorcluster, "Data out"=w381:u32[], "refnum out"=w377:refnum<file>, "EOF?"=w382:bool)  [unwired: 4 in]
                      n188 = Array Size(array=w381) -> (size(s)=w380:i32)
                      n189 = call "MTS_ToImageOffline.vi"("Data In"=w381, "Reset"=w379, "Image Array In"=w373, "Data Count"=w380) -> ("Image Array Out"=w375:i32[][], "Histograms"=w376:i32[][], "Traces"=w372:i32[][])  [unwired: 2 in, 7 out]
                    }
                    n190 = local write "Image"(w368) -> ()
                  }
                  frame "Point Measurement", Default {
                    w396 = TRUE ("Start From Top")
                    n191 = call "PT3_Read.vi"("Start From Top"=w396, "error in"=w395, "Data count"=10000, "refnum in"=w394) -> ("error out"=w389:errorcluster, "Data out"=w387:u32[], "refnum out"=w390:refnum<file>)  [unwired: 4 in, 1 out]
                    n192 = Array Size(array=w387) -> (size(s)=w386:i32)
                    n193 = call "MTS_ToImageOffline.vi"("Data In"=w387, "Reset"=w396, "Image Array In"=w393, "Data Count"=w386) -> ("Histograms"=w392:i32[][], "Traces"=w391:i32[][])  [unwired: 2 in, 8 out]
                  }
                }
                n194 = local write "Histogram"(w342) -> ()
                n195 = local write "Trace"(w341) -> ()
                n196 = Close File(refnum=w340, error in=w339) -> (error out=w338:errorcluster)  [unwired: 1 out]
              }
            }
          }
        }
      }
      event "x-Pixel", "Picture size", "y-Pixel", "Picture size 2": Value Change {
        w399 = 1000.0 ("y")
        n197 = event-data() -> ()  [unwired: 1 in, 5 out]
        n198 = local read "Picture size 2"() -> (w401:dbl)
        n199 = local read "Picture size"() -> (w405:dbl)
        n200 = local read "x-Pixel"() -> (w404:u16)
        n201 = local read "y-Pixel"() -> (w400:u16)
        n202 = Divide(x=w405, y=w404) -> (x/y=w403:dbl)
        n203 = Divide(x=w401, y=w400) -> (x/y=w402:dbl)
        n204 = Multiply(x=w403, y=w399) -> (x*y=→"x":dbl)
        n205 = Multiply(x=w402, y=w399) -> (x*y=→"y":dbl)
      }
      event "Excitation": Mouse Up {
        n206 = event-data() -> ()  [unwired: 1 in, 7 out]
        n207 = local read "MeasRunig"() -> (w407:bool)
        n208 = Not(x=w407) -> (.not. x?=w406:bool)
        n209 = case shown="True" w406 {
          frame False {
          }
          frame True {
            n210 = local read "Excitation"() -> (w411:bool)
            n211 = local read "Detector1"() -> (w409:bool)
            n212 = local read "Detector2"() -> (w408:bool)
            n213 = Not(x=w411) -> (.not. x?=w410:bool)
            n214 = call "PCAN_CompMessage.vi"("Detector2"=w408, "Detector1"=w409, "Excitation"=w410) -> ("CAN_Message"=w412:T21)
            n215 = call "CAN USB Write.vi"("CAN_Message"=w412) -> ()  [unwired: 2 in, 1 out]
          }
        }
      }
      event "Detector1": Mouse Up {
        n216 = event-data() -> ()  [unwired: 1 in, 7 out]
        n217 = local read "MeasRunig"() -> (w414:bool)
        n218 = Not(x=w414) -> (.not. x?=w413:bool)
        n219 = case shown="True" w413 {
          frame False {
          }
          frame True {
            n220 = local read "Excitation"() -> (w415:bool)
            n221 = local read "Detector1"() -> (w417:bool)
            n222 = local read "Detector2"() -> (w418:bool)
            n223 = Not(x=w417) -> (.not. x?=w416:bool)
            n224 = call "PCAN_CompMessage.vi"("Detector2"=w418, "Detector1"=w416, "Excitation"=w415) -> ("CAN_Message"=w419:T21)
            n225 = call "CAN USB Write.vi"("CAN_Message"=w419) -> ()  [unwired: 2 in, 1 out]
          }
        }
      }
      event "Detector2": Mouse Up {
        n226 = event-data() -> ()  [unwired: 1 in, 7 out]
        n227 = local read "MeasRunig"() -> (w421:bool)
        n228 = Not(x=w421) -> (.not. x?=w420:bool)
        n229 = case shown="True" w420 {
          frame False {
          }
          frame True {
            n230 = local read "Excitation"() -> (w425:bool)
            n231 = local read "Detector1"() -> (w424:bool)
            n232 = local read "Detector2"() -> (w422:bool)
            n233 = Not(x=w422) -> (.not. x?=w423:bool)
            n234 = call "PCAN_CompMessage.vi"("Detector2"=w423, "Detector1"=w424, "Excitation"=w425) -> ("CAN_Message"=w426:T21)
            n235 = call "CAN USB Write.vi"("CAN_Message"=w426) -> ()  [unwired: 2 in, 1 out]
          }
        }
      }
    }
    n236 = flat-sequence {
      tunnel: [w115] -> w112
      tunnel: w111 -> [w115]
      frame #0 {
      }
    }
    n237 = local read "Global Stop"() -> (w110:bool)
  }
  n238 = while {
    shift-right: [w432] -> w18
    shift-left: w20 -> [w427]
    tunnel: w22 -> [w440]
    tunnel: [w439] -> w26
    shift-right: [w434] -> w4
    shift-left: w23 -> [w441]
    tunnel: w19 -> [w433]
    shift-right: [w430] -> w2
    shift-left: w1 -> [w429]
    stop <- w437 stop-if-true
    n239 = case shown="No Error" w427 {
      selector: w427 -> [w443 w1032]
      tunnel: w441 -> [w457 w1030]
      tunnel: w440 -> [w456 w1031]
      tunnel: [w455 w1031] -> w439
      tunnel: [w454 TRUE ("Global Stop")] -> w436
      tunnel: [w450 w1030] -> w435
      tunnel: w433 -> [w449 _]
      tunnel: [w448 w1032] -> w432
      tunnel: [w446 w1029] -> w430
      tunnel: w429 -> [w445 w1029]
      tunnel: [w444 T3."No Measurement" ("Do Measurement")] -> w428
      frame No Error {
        # "Wait for Start"
        n240 = while {
          shift-right: [w1026] -> w451
          shift-left: w457 -> [w1026]
          tunnel: [w1023] -> w453
          tunnel: [w1022] -> w452
          tunnel: [w1021] -> w447
          stop <- w1027 stop-if-true
          w1021 = FALSE ("FiFo Overrun")
          n241 = local read "Do Measurement"() -> (w1023:T3)
          n242 = local read "Global Stop"() -> (w1022:bool)
          n243 = Wait (ms)(milliseconds to wait=u32 100) -> ()  [unwired: 1 out]
          n244 = local write "Stop Measurement"(w1021) -> ()
          n245 = Greater Than 0?(x=w1023) -> (x > 0?=w1025:bool)
          n246 = Or(x=w1025, y=w1022) -> (x .or. y?=w1027:bool)
        }
        n247 = control-ref of="WS File Tree"() -> (w442:refnum<vi>)
        n248 = local write "FiFo Overrun"(w447) -> ()
        n249 = case shown="\"Find Single Mol.\"" w453 {
          selector: w453 -> [_ _ w675 _ _ _ _]
          tunnel: w443 -> [w462 w540 w726 w831 w846 w921 w989]
          tunnel: w456 -> [w463 w539 w689 w832 w842 w917 w988]
          tunnel: [w463 w506 w678 w824 w842 w917 w988] -> w455
          tunnel: [w462 w514 w715 w825 w845 w920 w989] -> w448
          tunnel: [w461 FALSE ("Global Stop") FALSE ("Global Stop") FALSE ("Global Stop") FALSE ("Global Stop") FALSE ("Global Stop") FALSE ("Global Stop")] -> w454
          tunnel: w452 -> [w461 _ _ _ _ _ _]
          tunnel: w451 -> [w460 w501 w707 w823 w844 w919 w984]
          tunnel: [w460 w515 w716 w823 w844 w919 w980] -> w450
          tunnel: w449 -> [_ w536 w723 _ _ _ _]
          tunnel: w445 -> [w459 w466 w676 w821 w834 w905 w973]
          tunnel: [w459 w466 w676 w821 w834 w904 w972] -> w446
          tunnel: [T3."No Measurement" ("Do Measurement") T3."No Measurement" ("Do Measurement") w672 T3."No Measurement" ("Do Measurement") T3."No Measurement" ("Do Measurement") T3."No Measurement" ("Do Measurement") w979] -> w444
          tunnel: w442 -> [_ _ w654 _ _ _ _]
          frame "No Measurement", Default {
          }
          frame "Aquire Image" {
            w467 = T19."Image File" ("Measurement Type")
            w513 = 32768 ("dimension size")
            # "TODO:\n- FIFO Read Flag Buffer Half Full?\n- auto square pixels"
            # "Image Intensity Array"
            n250 = control-ref of="Image"() -> (w480:refnum<vi>)
            n251 = Bundle("X-Position"="X-Position", "Y-Position"="Y-Position", "Z-Position"="Z-Position") -> (w476:T22)  [unwired: 1 in]
            n252 = Build Array("x-Pixel", "y-Pixel") -> (w474:u16[])
            n253 = Cluster To Array(cluster=w476) -> (array=w538:dbl[])
            n254 = call "PI_Scanner_In_Range.vi"("Picture size"="Picture size", "Picture size 2"="Picture size 2", "Upper Left"=w476, "Axis"="Axis") -> ("Picture size out"=w500:dbl, "Picture size out 2"=w499:dbl)  [unwired: 14 in]
            n255 = call "PI_MoveTo.vi"("System no."=w539, "Target position"=w538, "error in"=w540, "Move"=TRUE) -> ("System no. (dup)"=w522:i32, "error out"=w479:errorcluster)  [unwired: 13 in, 1 out]
            n256 = Build Array(w500, w499) -> (w475:dbl[])
            n257 = Multiply(x="Scanner Divider", y=2.0) -> (x*y=w469:dbl)
            n258 = call "MTS_SetGraphScales.vi"("Pixels"=w474, "Axis"="Axis", "Picture Size"=w475, "error in (no error)"=w479, "Upper Left"=w476, "Image"=w480) -> ("error out"=w477:errorcluster)  [unwired: 5 in]
            n259 = call "MTS_GenFileComment.vi"("Time Per Pixel [ms]"=w469, "Measurement Type"=w467, "error in"=w501, "Upper Left"=w476, "Pixels"=w474, "Picture Size"=w475) -> ("error out"=w496:errorcluster, "Image Header"=w468:T23, "Image Info"=w486:T24, "Comment"=w498:string)  [unwired: 2 in]
            n260 = local read "Workspace"() -> (w497:path)
            n261 = control-ref of="WS File Tree"() -> (w485:refnum<vi>)
            n262 = call "PI_Image_Scanner_Prepare_Dlg.vi"("System no."=w522, "Picture Size"=w475, "Pixels"=w474, "Axis"="Axis", "Scanner Divider"="Scanner Divider", "error in"=w477, "Learning loop"="Learning loop") -> ("System no. (dup)"=w521:i32, "Measurement time [s]"=w518:i32, "error out"=w523:errorcluster)  [unwired: 6 in]
            n263 = local write "Picture size"(w500) -> ()
            n264 = local write "Picture size 2"(w499) -> ()
            n265 = Index Array(array=w536) -> (element=w535:T25)  [unwired: 1 in]
            n266 = call "MTS_GetNextFileName.vi"("error in (no error)"=w496, "File Type"="pt3", "Measurement Type"="Image", "Workspace"=w497) -> ("error out"=w489:errorcluster, "Next File Name"=w488:path)  [unwired: 6 in]
            n267 = Unbundle By Name(w535) -> ("Dev"=w532:i32)
            n268 = call "PH_Set.vi"("Device List"=w536, "error in (no error)"=w523) -> ("pt3 header out"=w503:T26, "Count Rate"=w525:i32, "error out"=w505:errorcluster)  [unwired: 8 in, 3 out]
            n269 = Initialize Array(0 ("element"), "x-Pixel", "y-Pixel") -> (w526:i32[][])
            n270 = call "MTS_AddFileToWorkspace.vi"("File Name"=w488, "File Type"=T14."pt3 File", "Scan Axis"="Axis", "Measurement Type"=w467, "File Info"=w486, "error in (no error)"=w489, "Tree Refnum"=w485) -> ("File Name (dup)"=w473:path, "File No"=→"Last Image File No":i32, "error out"=w487:errorcluster)  [unwired: 6 in]
            n271 = call "MTS_CalcMeasTime.vi"("Scanner Divider"="Scanner Divider", "pt3 header in"=w503, "Measurement time [s]"=w518, "Count Rate"=w525) -> ("pt3 header out"=w502:T26, "Corrected Measurement time [s]"=→"Measure. time [s]":i32, "Calc Acq. Time (ms)"=w529:i32, "Overflow Interv. Time (s)"=w528:dbl, "Pixel Time (Laser Pulses)"=w524:i32)  [unwired: 7 in]
            n272 = call "PT3_Create.vi"("Image Header in"=w468, "Save pt3"="Save Files", "Measurement Type"=w467, "error in"=w505, "Comment"=w498, "pt3 Header in"=w502, "File Path"=w473) -> ("error out"=w504:errorcluster, "refnum out"=w493:refnum<file>)  [unwired: 3 in]
            n273 = call "PH_Start.vi"("Device Index"=w532, "Acq. Time"=w529, "error in (no error)"=w504) -> ("error out"=w533:errorcluster)  [unwired: 11 in, 1 out]
            n274 = local write "Active pt3"(w473) -> ()
            n275 = To Unsigned Long Integer(number=w513) -> (unsigned 32bit integer=w510:u32)
            n276 = Initialize Array(u32 0, w513) -> (w511:u32[])
            n277 = Unbundle By Name(w533) -> ("status"=w534:bool)
            n278 = Not(x=w534) -> (.not. x?=w531:bool)
            n279 = case shown="True" w531 {
              tunnel: [w594 w621] -> w516
              tunnel: [w596 w613] -> w507
              tunnel: w521 -> [w596 w610]
              tunnel: w533 -> [w595 w611]
              tunnel: w487 -> [w597 w619]
              tunnel: [w597 w618] -> w517
              tunnel: w532 -> [w593 w620]
              tunnel: w528 -> [_ w600]
              tunnel: w526 -> [_ w615]
              tunnel: w524 -> [_ w614]
              tunnel: "Axis" -> [_ w609]
              tunnel: w511 -> [_ w608]
              tunnel: w510 -> [_ w607]
              tunnel: [w592 w606] -> w509
              tunnel: [w592 w605] -> w508
              tunnel: w493 -> [w591 w604]
              tunnel: [w591 w603] -> w492
              tunnel: [0 ("Num Records Total") w602] -> w491
              tunnel: [0.0 w599] -> w490
              tunnel: [u64[] [] ("Histograms") w598] -> w484
              frame False {
                w592 = FALSE ("Stop Measurement")
                n280 = call "PH_Stop.vi"("Device Index"=w593, "error in (no error)"=w595) -> ("error out"=w594:errorcluster)  [unwired: 12 in, 1 out]
              }
              frame True {
                # "Overflow Interv. Time (s)"
                # "No Error"
                n281 = call "PI_Start_Wave_Gen.vi"("System no."=w610, "error in"=w611, "Axis"=w609) -> ("System no. (dup)"=w613:i32, "error out"=w612:errorcluster)  [unwired: 11 in]
                n282 = while {
                  tunnel: w620 -> [w649]
                  tunnel: w608 -> [w648]
                  tunnel: w607 -> [w647]
                  shift-right: [w633] -> w617
                  shift-left: w612 -> [w650]
                  shift-right: [w646] -> w618
                  shift-left: w619 -> [w646]
                  shift-right: [FALSE ("Reset")] -> _
                  shift-left: TRUE ("Reset") -> [w642]
                  tunnel: w615 -> [w639]
                  tunnel: w614 -> [w635]
                  tunnel: [w636] -> w606
                  tunnel: [w626] -> w605
                  tunnel: w604 -> [w630]
                  tunnel: [w629] -> w603
                  tunnel: [w628] -> w602
                  tunnel: [w627] -> w601
                  tunnel: [w622] -> w598
                  stop <- w645 stop-if-true
                  n283 = call "PH_FIFORead.vi"("Device Index"=w649, "Buffer In"=w648, "Count"=w647, "error in (no error)"=w650) -> ("OK"=w637:bool, "Buffer Out"=w631:u32[], "Data Count"=w632:i32, "FiFo Overrun"=w636:bool, "error out"=w634:errorcluster)  [unwired: 7 in]
                  n284 = local write "FiFo Overrun"(w636) -> ()
                  n285 = local read "Global Stop"() -> (w624:bool)
                  n286 = Wait (ms)(milliseconds to wait=u32 10) -> ()  [unwired: 1 out]
                  n287 = Unbundle(w634) -> ("status"=w644:bool)  [unwired: 2 out]
                  n288 = call "PH_ToImage.vi"("Data In"=w631, "Reset"=w642, "Image Array In"=w639, "Data Count"=w632, "Pixel Time (Laser Pulses)"=w635) -> ("Image Array Out"=→"Image":i32[][], "Histograms"=→"Histogram":i32[][], "Total Photon Count"=w622:u64[], "Total Oveflow Count"=w627:u64, "Num Records Total"=w628:i32, "Traces"=→"Trace":i32[][])  [unwired: 4 in, 1 out]
                  n289 = local read "Stop Measurement"() -> (w625:bool)
                  n290 = call "PT3_Write.vi"("error in"=w634, "Data Count"=w632, "Data in"=w631, "refnum in"=w630) -> ("error out"=w633:errorcluster, "refnum out"=w629:refnum<file>)  [unwired: 6 in]
                  n291 = Compound Arithmetic op=OR(invert w637, w644, w624, w625) -> (w645:bool)
                  n292 = Or(x=w625, y=w624) -> (x .or. y?=w626:bool)
                }
                n293 = Multiply(x=w600, y=w601) -> (x*y=w599:dbl)
                n294 = call "PH_Stop.vi"("Device Index"=w620, "error in (no error)"=w617) -> ("error out"=w621:errorcluster)  [unwired: 12 in, 1 out]
              }
            }
            n295 = control-ref of="WS File Tree"() -> (w482:refnum<vi>)
            n296 = flat-sequence {
              tunnel: w517 -> [w576]
              tunnel: w516 -> [w572]
              tunnel: [w576] -> w515
              tunnel: [w550] -> w514
              tunnel: w509 -> [w574]
              tunnel: w508 -> [w561]
              tunnel: w507 -> [w571]
              tunnel: [w570] -> w506
              tunnel: w492 -> [w567]
              tunnel: w491 -> [w566]
              tunnel: w490 -> [w559]
              tunnel: w484 -> [w560]
              tunnel: "Save Files" -> [w549]
              tunnel: w473 -> [w548]
              tunnel: w482 -> [w547]
              frame #0 {
                # "Count Rate (per s)"
                # "Stop WaveGen\nif Aborted"
                # "Finish after Aquire Image"
                n297 = Or(x=w561, y=w574) -> (x .or. y?=w573:bool)
                n298 = case shown="False" w573 {
                  tunnel: w572 -> [w579 w587]
                  tunnel: w571 -> [w578 w586]
                  tunnel: [w578 w585] -> w570
                  tunnel: [w579 w584] -> w568
                  tunnel: [enum16{"timeover", "manual", "overflow"}."timeover" ("Stop Reason") w582] -> w562
                  tunnel: w561 -> [_ w580]
                  frame False {
                  }
                  frame True {
                    n299 = call "PI_Stop_Wave_Gen.vi"("System no."=w586, "error in"=w587) -> ("System no. (dup)"=w585:i32, "error out"=w584:errorcluster)  [unwired: 12 in]
                    n300 = Select(t=enum16{"timeover", "manual", "overflow"}."manual" ("Stop Reason"), s=w580, f=enum16{"timeover", "manual", "overflow"}."overflow" ("Stop Reason")) -> (s? t:f=w582:enum16{"timeover", "manual", "overflow"})
                  }
                }
                n301 = Multiply(x=w559, y=1000.0) -> (x*y=w564:dbl)
                n302 = Divide(x=w560, y=w559) -> (x/y=w558:dbl[])
                n303 = To Long Integer(number=w564) -> (32bit integer=w563:i32)
                n304 = To Long Integer(number=w558) -> (32bit integer=w557:i32[])
                n305 = property on="Aquire Image" class="Bool"("BoolText.Text"="Aquire Image" ("Caption.Text"), "BoolText.TextColor"=u32 0 ("Boolean Text.Colors:FG Color")) -> ()  [unwired: 2 in, 2 out]
                n306 = Index Array(array=w557, index #1=0 ("index"), index #2=1 ("index")) -> (element #1=w554:i32, element #2=w553:i32)
                n307 = local read "Image"() -> (w552:i32[][])
                n308 = call "PT3_Finish.vi"("Input 1 Rate"=w553, "Input 0 Rate"=w554, "Stop Reason"=w562, "error in"=w568, "Num Records"=w566, "Stop After (ms)"=w563, "refnum in"=w567) -> ("error out"=w551:errorcluster)  [unwired: 4 in]
                n309 = call "MTS_SaveImagePng.vi"("Save .png"=w549, "Tree Refnum"=w547, ".pt3 File Name"=w548, "error in"=w551, "Image"=w552) -> ("error out"=w550:errorcluster)  [unwired: 6 in]
              }
            }
          }
          frame "Point Measurement", "Auto Point" {
            w714 = 32768 ("dimension size")
            n310 = local read "Workspace"() -> (w705:path)
            n311 = local read "X-Position"() -> (w692:dbl)
            n312 = local read "Y-Position"() -> (w691:dbl)
            n313 = local read "Z-Position"() -> (w690:dbl)
            n314 = local read "Pattern"() -> (w656:dbl[][])
            n315 = local read "NxtAutMesPoint"() -> (w655:i32)
            n316 = local read "Last Image File No"() -> (w661:i32)
            n317 = Index Array(array=w723) -> (element=w722:T25)  [unwired: 1 in]
            n318 = Bundle("X-Position"=w692, "Y-Position"=w691, "Z-Position"=w690) -> (w658:T22)  [unwired: 1 in]
            n319 = Equal?(x=w675, y=T3."Auto Point" ("Do Measurement")) -> (x = y?=w652:bool)
            n320 = Unbundle By Name(w722) -> ("Dev"=w679:i32)
            n321 = call "MTS_AutoPointCords.vi"("Is Auto Point"=w652, "Cords In"=w658, "Next Auto Measure Point"=w655, "Pattern"=w656) -> ("Cords"=w657:T22)  [unwired: 7 in]
            n322 = Cluster To Array(cluster=w657) -> (array=w725:dbl[])
            n323 = Select(t="Auto Measurement Time (ms)", s=w652, f="Measurement Time (ms)") -> (s? t:f=w662:i32)
            n324 = call "PI_MoveTo.vi"("System no."=w689, "Target position"=w725, "error in"=w726, "Move"=TRUE) -> ("System no. (dup)"=w678:i32, "error out"=w693:errorcluster)  [unwired: 13 in, 1 out]
            n325 = Select(t="AutoPoint" ("Measurement Type"), s=w652, f="Point" ("Measurement Type")) -> (s? t:f=w665:string)
            n326 = Select(t=T19."Auto Point" ("Measurement Type"), s=w652, f=T19."Point Measurement" ("Measurement Type")) -> (s? t:f=w666:T19)
            n327 = Select(t=w661, s=w652, f=-1) -> (s? t:f=w659:i32)
            n328 = call "MTS_GenFileComment.vi"("Parent File No"=w659, "Measurement Type"=w666, "error in"=w707, "Upper Left"=w657) -> ("error out"=w704:errorcluster, "Image Info"=w694:T24, "Comment"=w706:string)  [unwired: 4 in, 1 out]
            n329 = call "PH_Set.vi"("Device List"=w723, "error in (no error)"=w693) -> ("pt3 header out"=w685:T26, "Count Rate"=w686:i32, "error out"=w681:errorcluster)  [unwired: 8 in, 3 out]
            n330 = Bundle By Name(cluster=w685, "AcquisitionTime (ms)"=w662) -> (w684:T26)
            n331 = And(x=w652, y="Autopoint-Auto Z") -> (x .and. y?=w651:bool)
            n332 = Reciprocal(x=w686) -> (1/x=w688:dbl)
            n333 = call "MTS_GetNextFileName.vi"("error in (no error)"=w704, "File Type"="pt3", "Measurement Type"=w665, "Workspace"=w705) -> ("error out"=w698:errorcluster, "Next File Name"=w697:path)  [unwired: 6 in]
            n334 = Scale By Power Of 2(n=16, x=w688) -> (x*2^n=w677:dbl)
            n335 = case shown="True" w651 {
              tunnel: w681 -> [w728 w736]
              tunnel: [w728 w735] -> w680
              tunnel: w679 -> [_ w734]
              tunnel: w678 -> [_ w733]
              tunnel: w677 -> [_ w732]
              tunnel: w657 -> [_ w731]
              frame False {
              }
              frame True {
                # "Auto Z"
                n336 = call "MTS_AutoZPos.vi"("PH Dev"=w734, "OFlow Interv [s]"=w732, "PI System no."=w733, "error in"=w736, "Start Point"=w731) -> ("New Z"=w730:dbl, "Counts"=→"Counts":u32[], "error out"=w735:errorcluster)  [unwired: 8 in]
                n337 = local write "Z-Position"(w730) -> ()
              }
            }
            n338 = call "MTS_AddFileToWorkspace.vi"("File Name"=w697, "File Type"=T14."pt3 File", "Measurement Type"=w666, "File Info"=w694, "error in (no error)"=w698, "Parent"=w659, "Tree Refnum"=w654) -> ("File Name (dup)"=w695:path, "error out"=w696:errorcluster)  [unwired: 6 in, 1 out]
            n339 = call "PT3_Create.vi"("error in"=w680, "Comment"=w706, "pt3 Header in"=w684, "File Path"=w695) -> ("error out"=w708:errorcluster, "refnum out"=w702:refnum<file>)  [unwired: 6 in]
            n340 = call "PH_Start.vi"("Device Index"=w679, "Acq. Time"=w662, "error in (no error)"=w708) -> ("error out"=w720:errorcluster)  [unwired: 11 in, 1 out]
            n341 = To Unsigned Long Integer(number=w714) -> (unsigned 32bit integer=w711:u32)
            n342 = Initialize Array(u32 0, w714) -> (w712:u32[])
            n343 = Unbundle By Name(w720) -> ("status"=w721:bool)
            n344 = Not(x=w721) -> (.not. x?=w719:bool)
            n345 = case shown="True" w719 {
              tunnel: [w773 w793] -> w717
              tunnel: w720 -> [w774 w777]
              tunnel: w696 -> [w775 w791]
              tunnel: [w775 w790] -> w718
              tunnel: w679 -> [w772 w792]
              tunnel: w677 -> [_ w779]
              tunnel: w712 -> [_ w787]
              tunnel: w711 -> [_ w786]
              tunnel: [w771 w785] -> w710
              tunnel: [w771 w784] -> w709
              tunnel: w702 -> [w770 w783]
              tunnel: [w770 w782] -> w701
              tunnel: [0 ("Num Records Total") w781] -> w700
              tunnel: [0.0 w778] -> w699
              tunnel: [u64[] [] ("Total Photon Count") w776] -> w683
              frame False {
                w771 = FALSE ("Stop Measurement")
                n346 = call "PH_Stop.vi"("Device Index"=w772, "error in (no error)"=w774) -> ("error out"=w773:errorcluster)  [unwired: 12 in, 1 out]
              }
              frame True {
                # "Overflow Interv. Time (s)"
                # "No Error"
                n347 = while {
                  tunnel: w792 -> [w818]
                  tunnel: w787 -> [w817]
                  tunnel: w786 -> [w816]
                  shift-right: [w806] -> w789
                  shift-left: w777 -> [w819]
                  shift-right: [w815] -> w790
                  shift-left: w791 -> [w815]
                  shift-right: [FALSE ("Reset")] -> _
                  shift-left: TRUE ("Reset") -> [w811]
                  tunnel: [w808] -> w785
                  tunnel: [w799] -> w784
                  tunnel: w783 -> [w803]
                  tunnel: [w802] -> w782
                  tunnel: [w801] -> w781
                  tunnel: [w800] -> w780
                  tunnel: [w794] -> w776
                  stop <- w814 stop-if-true
                  n348 = call "PH_FIFORead.vi"("Device Index"=w818, "Buffer In"=w817, "Count"=w816, "error in (no error)"=w819) -> ("OK"=w809:bool, "Buffer Out"=w804:u32[], "Data Count"=w805:i32, "FiFo Overrun"=w808:bool, "error out"=w807:errorcluster)  [unwired: 7 in]
                  n349 = local write "FiFo Overrun"(w808) -> ()
                  n350 = local read "Global Stop"() -> (w797:bool)
                  n351 = Wait (ms)(milliseconds to wait=u32 10) -> ()  [unwired: 1 out]
                  n352 = Unbundle(w807) -> ("status"=w813:bool)  [unwired: 2 out]
                  n353 = call "PH_TraceAndHisto.vi"("Data In"=w804, "Reset"=w811, "Data Count"=w805) -> ("Histograms"=w796:i32[][], "Total Photon Count"=w794:u64[], "Total Oveflow Count"=w800:u64, "Num Records Total"=w801:i32, "Traces"=w795:i32[][])  [unwired: 8 in]
                  n354 = local read "Stop Measurement"() -> (w798:bool)
                  n355 = call "PT3_Write.vi"("error in"=w807, "Data Count"=w805, "Data in"=w804, "refnum in"=w803) -> ("error out"=w806:errorcluster, "refnum out"=w802:refnum<file>)  [unwired: 6 in]
                  n356 = local write "Histogram"(w796) -> ()
                  n357 = local write "Trace"(w795) -> ()
                  n358 = Compound Arithmetic op=OR(invert w809, w813, w797, w798) -> (w814:bool)
                  n359 = Or(x=w798, y=w797) -> (x .or. y?=w799:bool)
                }
                n360 = Multiply(x=w779, y=w780) -> (x*y=w778:dbl)
                n361 = call "PH_Stop.vi"("Device Index"=w792, "error in (no error)"=w789) -> ("error out"=w793:errorcluster)  [unwired: 12 in, 1 out]
              }
            }
            n362 = flat-sequence {
              tunnel: w718 -> [w759]
              tunnel: w717 -> [w755]
              tunnel: [w759] -> w716
              tunnel: [w752] -> w715
              tunnel: w710 -> [w757]
              tunnel: w709 -> [w745]
              tunnel: w701 -> [w751]
              tunnel: w700 -> [w750]
              tunnel: w699 -> [w740]
              tunnel: w683 -> [w739]
              frame #0 {
                # "Finish after Measurement"
                n363 = Or(x=w745, y=w757) -> (x .or. y?=w756:bool)
                n364 = case shown="True" w756 {
                  tunnel: w755 -> [w761 w762]
                  tunnel: [w761 w762] -> w753
                  tunnel: [enum16{"timeover", "manual", "overflow"}."timeover" ("Stop Reason") w765] -> w746
                  tunnel: w745 -> [_ w763]
                  frame False {
                  }
                  frame True {
                    n365 = Select(t=enum16{"timeover", "manual", "overflow"}."manual" ("Stop Reason"), s=w763, f=enum16{"timeover", "manual", "overflow"}."overflow" ("Stop Reason")) -> (s? t:f=w765:enum16{"timeover", "manual", "overflow"})
                  }
                }
                n366 = Multiply(x=w740, y=1000.0) -> (x*y=w748:dbl)
                n367 = Divide(x=w739, y=w740) -> (x/y=w741:dbl[])
                n368 = To Long Integer(number=w748) -> (32bit integer=w747:i32)
                n369 = To Long Integer(number=w741) -> (32bit integer=w742:i32[])
                n370 = property on="Point Measurement" class="Bool"("BoolText.Text"="Point Measurement" ("Caption.Text"), "BoolText.TextColor"=u32 0 ("Boolean Text.Colors:FG Color")) -> ()  [unwired: 2 in, 2 out]
                n371 = Index Array(array=w742, index #1=0 ("index"), index #2=1 ("index")) -> (element #1=w738:i32, element #2=w737:i32)
                n372 = call "PT3_Finish.vi"("Input 1 Rate"=w737, "Input 0 Rate"=w738, "Stop Reason"=w746, "error in"=w753, "Num Records"=w750, "Stop After (ms)"=w747, "refnum in"=w751) -> ("error out"=w752:errorcluster)  [unwired: 4 in]
              }
            }
            n373 = Select(t=T3."Auto Measurement Control" ("Do Measurement"), s=w652, f=T3."No Measurement" ("Do Measurement")) -> (s? t:f=w672:T3)
          }
          frame "Multi Measurement" {
            n374 = local read "X-Position"() -> (w830:dbl)
            n375 = local read "Y-Position"() -> (w829:dbl)
            n376 = local read "Z-Position"() -> (w828:dbl)
            n377 = Build Array(w830, w829, w828) -> (w827:dbl[])
            n378 = call "PI_MoveTo.vi"("System no."=w832, "Target position"=w827, "error in"=w831, "Move"=TRUE) -> ("System no. (dup)"=w824:i32, "error out"=w825:errorcluster)  [unwired: 13 in, 1 out]
          }
          frame "Save Color Image" {
            n379 = local read "Active pt3"() -> (w840:path)
            n380 = call "MTS_GetFileFromWS.vi"(".pt3 File Name"=w840) -> ("File Header"=w839:T18)  [unwired: 9 in, 1 out]
            n381 = Unbundle By Name(w839) -> ("Measurement Type"=w838:T19, "Pixels"=w835:i32[])
            n382 = Equal?(x=T19."Image File" ("Measurement Type"), y=w838) -> (x = y?=w836:bool)
            n383 = control-ref of="WS File Tree"() -> (w841:refnum<vi>)
            n384 = case shown="True" w836 {
              tunnel: w846 -> [w847 w876]
              tunnel: w840 -> [_ w875]
              tunnel: w840 -> [_ w858]
              tunnel: [w847 w848] -> w845
              tunnel: w841 -> [_ w855]
              tunnel: w835 -> [_ w854]
              frame False {
              }
              frame True {
                # "Image Intensity Array"
                # "Image Intensity Array"
                n385 = call "PT3_Open.vi"("error in"=w876, "File Path"=w875) -> ("error out"=w868:errorcluster, "Header"=w872:T27, "refnum out"=w874:refnum<file>)  [unwired: 3 in, 4 out]
                n386 = Index Array(array=w854, index #2=1 ("index")) -> (element #1=w851:i32, element #2=w852:i32)  [unwired: 1 in]
                n387 = Unbundle By Name(w872) -> ()  [unwired: 15 out]
                n388 = Initialize Array(0 ("element"), w851, w852) -> (w870:i32[][])
                n389 = while {
                  tunnel: w874 -> [w902]
                  shift-right: [FALSE ("Start From Top")] -> _
                  shift-left: TRUE ("Start From Top") -> [w896]
                  shift-right: [w895] -> w867
                  shift-left: w868 -> [w890]
                  tunnel: [w894] -> w866
                  tunnel: w870 -> [w893]
                  tunnel: [w892] -> w869
                  tunnel: [w891] -> _
                  stop <- w899 stop-if-true
                  n390 = call "PT3_Read.vi"("Start From Top"=w896, "error in"=w890, "Data count"=10000, "refnum in"=w902) -> ("error out"=w895:errorcluster, "Data out"=w898:u32[], "refnum out"=w894:refnum<file>, "EOF?"=w899:bool)  [unwired: 4 in]
                  n391 = Array Size(array=w898) -> (size(s)=w897:i32)
                  n392 = call "MTS_ToImageOffline.vi"("Data In"=w898, "Reset"=w896, "Image Array In"=w893, "Data Count"=w897) -> ("Image Array Out"=w891:i32[][], "Histograms"=w892:i32[][])  [unwired: 2 in, 8 out]
                }
                n393 = call "MTS_SelectTCSPCBinning.vi"("Histograms in"=w869) -> ("TCSPC Binning"=w862:i32[][], "Colors"=w856:u32[], "Active"=w857:bool[])  [unwired: 1 in, 7 out]
                n394 = Initialize Array(0 ("element"), 4 ("dimension size"), w851, w852) -> (w863:i32[][][])
                n395 = while {
                  tunnel: w866 -> [w889]
                  shift-right: [FALSE ("Start From Top")] -> _
                  shift-left: TRUE ("Start From Top") -> [w883]
                  shift-right: [w882] -> w860
                  shift-left: w867 -> [w878]
                  tunnel: [w881] -> w849
                  tunnel: w863 -> [w880]
                  tunnel: [w879] -> w859
                  tunnel: w862 -> [w877]
                  stop <- w886 stop-if-true
                  n396 = call "PT3_Read.vi"("Start From Top"=w883, "error in"=w878, "Data count"=10000, "refnum in"=w889) -> ("error out"=w882:errorcluster, "Data out"=w885:u32[], "refnum out"=w881:refnum<file>, "EOF?"=w886:bool)  [unwired: 4 out]
                  n397 = Array Size(array=w885) -> (size(s)=w884:i32)
                  n398 = call "MTS_ToColorImage.vi"("Data In"=w885, "Reset"=w883, "Image Array In"=w880, "Data Count"=w884, "TCSPC Binning"=w877) -> ("Image Array Out"=w879:i32[][][])  [unwired: 2 in, 8 out]
                }
                n399 = call "MTS_SaveColorImagePng.vi"("Tree Refnum"=w855, ".pt3 File Name"=w858, "error in"=w860, "Colors"=w856, "Active"=w857, "Image"=w859) -> ("error out"=w850:errorcluster)  [unwired: 5 in]
                n400 = Close File(refnum=w849, error in=w850) -> (error out=w848:errorcluster)  [unwired: 1 out]
              }
            }
          }
          frame "Find Single Mol." {
            n401 = local read "Active pt3"() -> (w916:path)
            n402 = call "MTS_GetFileFromWS.vi"(".pt3 File Name"=w916) -> ("File Header"=w915:T18)  [unwired: 9 in, 1 out]
            n403 = Unbundle By Name(w915) -> ("Measurement Type"=w914:T19, "Pixels"=w911:i32[], "Picture Size"=w910:dbl[], "Upper Left"=w909:T20, "Scan Axis"=w908:enum32{"x-y", "x-z", "y-z"})
            n404 = call "MTS_ScannerXYZToImageXY.vi"("Axis"=w908, "Scanner XYZ"=w909) -> ("Image Y"=w906:dbl, "Image X"=w907:dbl)
            n405 = Equal?(x=T19."Image File" ("Measurement Type"), y=w914) -> (x = y?=w912:bool)
            n406 = case shown="True" w912 {
              tunnel: w921 -> [w923 w950]
              tunnel: w916 -> [_ _]
              tunnel: w916 -> [_ _]
              tunnel: [w923 w924] -> w920
              tunnel: w911 -> [_ w957]
              tunnel: w910 -> [_ w956]
              tunnel: w907 -> [_ w944]
              tunnel: w906 -> [_ w945]
              tunnel: w905 -> [w922 w938]
              tunnel: [w922 w933] -> w904
              frame False {
              }
              frame True {
                w955 = 1 ("index")
                # "Gauss Width"
                # "Pixel Size [um]"
                n407 = Index Array(array=w957, index #2=w955) -> (element #1=w953:i32, element #2=w948:i32)  [unwired: 1 in]
                n408 = Index Array(array=w956, index #2=w955) -> (element #1=w954:dbl, element #2=w947:dbl)  [unwired: 1 in]
                n409 = local read "Image"() -> (w937:i32[][])
                n410 = Divide(x=w954, y=w953) -> (x/y=w941:dbl)
                n411 = Divide(x=w947, y=w948) -> (x/y=w946:dbl)
                n412 = Reciprocal(x=w941) -> (1/x=w940:dbl)
                n413 = To Double Precision Float(number=w937) -> (double precision float=w949:dbl[][])
                n414 = Multiply(x=w940, y="psf width [um]") -> (x*y=w951:dbl)
                n415 = script code="mask = GenGauss2D(gw);\n[err, bim, cim, sim, yc, xc, bc, cc, sc, len, imm] = FindPatternCP(Image, mask, [], [], [], 1.5);\nxc = xc - 1;\nyc = yc - 1;"("??"=w950, "gw"=w951, "Image"=w949) -> ("??"=w939:errorcluster, "xc"=w928:dbl[], "yc"=w927:dbl[])
                n416 = Multiply(x=w941, y=w928) -> (x*y=w943:dbl[])
                n417 = Multiply(x=w927, y=w946) -> (x*y=w942:dbl[])
                n418 = Add(x=w944, y=w943) -> (x+y=w930:dbl[])
                n419 = Add(x=w942, y=w945) -> (x+y=w929:dbl[])
                n420 = call "MTS_IntensityArrayToImage.vi"(0:"Image"=w938, 1:"Image"=w937, "error in (no error)"=w939, "Log Scale"=TRUE) -> ("Image Out"=w934:T2, "error out"=w935:errorcluster)  [unwired: 10 in]
                n421 = for {
                  shift-right: [w964] -> w933
                  shift-left: w934 -> [w965]
                  tunnel: w928 -> [w963] mode=indexing
                  tunnel: w927 -> [w962] mode=indexing
                  shift-right: [w966] -> w925
                  shift-left: w935 -> [w967]
                  tunnel: u32 16738560 -> [w961]
                  tunnel: 3.0 ("x") -> [w960]
                  n422 = call "MTS_DrawCrossIMAQIamge.vi"("Image"=w965, "Size"=w960, "Color"=w961, "X"=w963, "Y"=w962, "error in (no error)"=w967) -> ("Image Out"=w964:T2, "error out"=w966:errorcluster)  [unwired: 8 in]
                }
                "AM image" <- w933
                n423 = Build Array(w930, w929, w928, w927) -> (→"Pattern":dbl[][])
                n424 = flat-sequence {
                  tunnel: w925 -> [w958]
                  tunnel: [w958] -> w924
                  frame #0 {
                    n425 = local write "ShowTab"(T1."Auto Measurement" ("ShowTab")) -> ()
                  }
                }
              }
            }
          }
          frame "Auto Measurement Control" {
            # "Init"
            n426 = local read "Pattern"() -> (w978:dbl[][])
            n427 = local read "NxtAutMesPoint"() -> (w971:i32)
            n428 = Index Array(array=w978, index (row)=0) -> (element=w985:dbl[])  [unwired: 1 in]
            n429 = Less Than 0?(x=w971) -> (x < 0?=w983:bool)
            n430 = case shown="True" w983 {
              tunnel: w985 -> [_ w1020]
              tunnel: w984 -> [w1011 w1015]
              tunnel: [w1011 w1014] -> w981
              tunnel: [w1010 w1012] -> w970
              frame False {
                n431 = local read "Auto Measure Points"() -> (w1010:i32)
              }
              frame True {
                n432 = Array Size(array=w1020) -> (size(s)=w1012:i32)
                "Auto Measure Points" <- w1012
                n433 = Number To Decimal String(number=w1012) -> (decimal integer string=w1017:string)  [unwired: 1 in]
                n434 = Concatenate Strings("Point 1 / " ("Caption.Text"), w1017) -> (w1016:string)
                n435 = property on="Auto Meas Progress" class="Slide (strict)"(error in=w1015, "Scale.Minimum"=0.0 ("Scale.Range:Minimum"), "Scale.Maximum"=w1012, "Value"=1 ("Auto Meas Progress"), "Caption.Text"=w1016) -> (error out=w1014:errorcluster)  [unwired: 1 in, 1 out]
              }
            }
            n436 = Increment(x=w971) -> (x+1=w969:i32)
            "NxtAutMesPoint" <- w969
            n437 = Greater Or Equal?(x=w969, y=w970) -> (x >= y?=w982:bool)
            n438 = Increment(x=w969) -> (x+1=w968:i32)
            n439 = Index Array(array=w978, index (row) #1=2 ("index (row)"), index (col) #1=w969, index (row) #2=3 ("index (row)"), index (col) #2=w969) -> (element #1=w975:dbl, element #2=w974:dbl)
            n440 = case shown="True" w982 {
              tunnel: w981 -> [w1000 w1009]
              tunnel: [w1006 w1009] -> w980
              tunnel: [T3."Auto Point" ("Do Measurement") T3."No Measurement" ("Do Measurement")] -> w979
              tunnel: w968 -> [w1001 _]
              tunnel: w975 -> [w998 _]
              tunnel: w974 -> [w997 _]
              tunnel: w973 -> [w994 w1007]
              tunnel: [w993 w1007] -> w972
              tunnel: w970 -> [w990 _]
              frame False {
                # "Prpare For Next Point"
                n441 = call "MTS_DrawCrossIMAQIamge.vi"("Image"=w994, "Size"=3.0 ("x"), "Color"=u32 6618880, "X"=w998, "Y"=w997, "error in (no error)"=w1000) -> ("Image Out"=w993:T2, "error out"=w999:errorcluster)  [unwired: 8 in]
                n442 = Number To Decimal String(number=w990) -> (decimal integer string=w991:string)  [unwired: 1 in]
                n443 = Number To Decimal String(number=w1001) -> (decimal integer string=w1003:string)  [unwired: 1 in]
                n444 = Concatenate Strings("Point " ("Caption.Text"), w1003, " / " ("Caption.Text"), w991) -> (w1002:string)
                n445 = property on="Auto Meas Progress" class="Slide (strict)"(error in=w999, "Value"=w1001, "Caption.Text"=w1002) -> (error out=w1006:errorcluster)  [unwired: 1 in, 1 out]
                n446 = local write "AM image"(w993) -> ()
              }
              frame True {
                # "No More Points"
              }
            }
          }
        }
      }
      frame Error {
      }
    }
    n447 = flat-sequence {
      tunnel: w435 -> [w1039]
      tunnel: [w1039] -> w434
      tunnel: w428 -> [w1035]
      frame #0 {
        n448 = control-ref of="ShowTab"() -> (w1038:refnum<vi>)
        n449 = Equal?(x=w1035, y=T3."No Measurement" ("Do Measurement")) -> (x = y?=w1034:bool)
        n450 = Not(x=w1034) -> (.not. x?=w1037:bool)
        n451 = case shown="True" w1034 {
          tunnel: w1038 -> [_ w1040]
          frame False {
          }
          frame True {
            n452 = call "MTS_ShowHideTabs.vi"("Action"=enum16{"Show All", "Hide Tab", "Show Tab"}."Show All", "ShowTab"=w1040) -> ()  [unwired: 8 in, 2 out]
          }
        }
        n453 = local write "Do Measurement"(w1035) -> ()
        n454 = local write "MeasRunig"(w1037) -> ()
      }
    }
    n455 = Unbundle(w432) -> ("status"=w431:bool)  [unwired: 2 out]
    n456 = local read "Global Stop"() -> (w438:bool)
    n457 = Compound Arithmetic op=OR(w431, w436, w438) -> (w437:bool)
  }
  n458 = while {
    tunnel: w22 -> [w1045]
    shift-right: [w1044] -> _
    shift-left: w21 -> [w1046]
    stop <- w1043 stop-if-true
    n459 = Wait (ms)(milliseconds to wait=u32 50) -> ()  [unwired: 1 out]
    n460 = case shown="True" "SCANNER EMERGENCY" {
      tunnel: w1045 -> [_ w1051]
      tunnel: w1046 -> [w1049 w1052]
      tunnel: [w1049 w1053] -> w1044
      frame False {
        n461 = Wait Until Next ms Multiple(millisecond multiple=u32 100) -> ()  [unwired: 1 out]
      }
      frame True {
        n462 = call "PI_Stop_Wave_Gen.vi"("System no."=w1051, "error in"=w1052) -> ("error out"=w1050:errorcluster)  [unwired: 12 in, 1 out]
        n463 = flat-sequence {
          tunnel: [w1054] -> w1053
          tunnel: w1050 -> [w1054]
          frame #0 {
            n464 = One Button Dialog(message="Emergency scanner stop appeared!!!\nCheck scanner settings before continue!!!") -> ()  [unwired: 2 out]
          }
        }
      }
    }
    n465 = local read "Global Stop"() -> (w1043:bool)
  }
  n466 = call "DT3120_CloseDevice.vi"("error in (no error)"=w15, "lpDevId"=w13) -> ("error out"=w8:errorcluster)  [unwired: 9 out]
  n467 = call "IMAQ Dispose"("Image"=w7, "error in (no error)"=w8) -> ("error out"=w6:errorcluster)  [unwired: 4 in]
  n468 = flat-sequence {
    tunnel: w6 -> [w1058]
    tunnel: [w1056] -> w5
    frame #0 {
      n469 = call "CAN USB Close.vi"() -> ("Error Number"=w1057:u32)  [unwired: 1 in]
      n470 = call <vilib>:"Error Cluster From Error Code.vi"("error in (no error)"=w1058, "error message (\"\")"="PCAN Close Error" ("error message (\"\")"), "error code (0)"=w1057) -> ("error out"=w1056:errorcluster)  [unwired: 6 in]
    }
  }
  n471 = Merge Errors(w5, w12) -> (w11:errorcluster)
  n472 = flat-sequence {
    tunnel: w18 -> [w1060]
    tunnel: [w1060] -> w17
    frame #0 {
      n473 = local write "Global Stop"(TRUE ("Global Stop")) -> ()
    }
  }
  n474 = call "IMAQ Dispose"("Image"=w2, "error in (no error)"=w4) -> ("error out"=w3:errorcluster)  [unwired: 4 in]
  n475 = call <userlib>:"Close connection if open.vi"("System no."=w26, "error in"=w17) -> ("error out"=w25:errorcluster)  [unwired: 16 in, 1 out]
  n476 = Merge Errors(w11, w3, w25) -> (w24:errorcluster)
  n477 = call <vilib>:"Simple Error Handler.vi"("error in (no error)"=w24) -> ()  [unwired: 4 in, 5 out]
